vi "PPMS Interface.vi"() -> ()   [LabVIEW 2020]
uses:
  <vilib>/Analysis/1siggen.llb/Ramp Pattern by Samples.vi
  <vilib>/Utility/file.llb/Write Delimited Spreadsheet (string).vi
  <vilib>/Utility/file.llb/Write Delimited Spreadsheet (DBL).vi
  <vilib>/Analysis/NI_AALBase.lvlib
panel:
  out "IV Data":dbl[][](array[numeric])
  in  "scan_npts":i16
  out "scan_points":dbl[](array[numeric])
  out "scan_RATE":dbl=20.0
  out "scan_counter":i16=1000
  out "scan_head":i32=55
  out "scan_new":bool caption="Scan New"
  out "scan_env":string="MEASURE"
  out "Seq Line Now":i32=55
  out "AC Flag":bool caption="AC Current"
  in  "Filetype":u16(ring)=2 items=[".xlsx", ".txt", ".csv"]
  out "Wait Done":dbl=10.0
  in  "Measurement setup tabs":enum32{"DC Setup", "AC Setup", "I-V Setup"}(tab)=enum."AC Setup"
  in  "DC Pulse":bool=TRUE caption="Current Pulsing"
  in  "Channel 2":bool
  in  "Channel 1":bool=TRUE
  in  "Current Amplitude":string="1e-4"
  in  "Time Period (s)":string="3"
  in  "Tpad(ms)":i32=200
  in  "Voltmeter Range (V)":string="0.01"
  in  "NPLC":string="1"
  in  "Voltmeter Buffer Size":string="62"
  in  "Voltmeter 2 Address":string="8"
  in  "Voltmeter 1 Address":string="7"
  in  "6221 Address":string="12"
  in  "Configure DC System":bool
  in  "6221 Address 2":string="12" caption="6221 Address"
  in  "Current Amplitude 2":string="1e-4" caption="Current \nAmplitude"
  in  "Ch2 Enable":bool
  in  "Ch1 Enable":bool=TRUE
  in  "Buffer Data":enum16{"X", "XY", "RT", "XYRT"}(ring)=enum."RT"
  in  "Rate decimation":i32=2
  in  "SR860 Ch2 Address":string="5"
  in  "SR860 Ch1 Address":string="4"
  in  "Frequency":string="1711"
  in  "Filter BW":T1(ring)=enum."100ms"
  in  "Ch1 Harmonic":T2(ring)
  in  "Buffer Size (kB)":i32=2
  in  "Configure AC System":bool
  in  "Buffer Offset (kb)":string="0"
  in  "Ch2 Harmonic":T2(ring)
  in  "IV Datafile Root":path=path "C:/Users/QDUser/Desktop/LabVIEW Programs/PPMS Interface/testfiles/data/DC_IV_test"
  in  "SR860 Address - IV":string="4" caption="SR860 Address"
  in  "6221 Address - IV":string="12" caption="6221 Address"
  in  "IV Sampling":enum16{"Linear", "Logartihmic"}(ring)=enum."Logartihmic"
  in  "IV Type":T3(ring)
  in  "dI or Imin":dbl=1e-08
  in  "Imax":dbl=0.0001
  in  "Points":i16=17
  in  "2182A Address - IV":string="7" caption="2182A Address"
  in  "IV - DC/AC":bool=TRUE
  in  "DC Period (s)":string="0.5" caption="6221 Address"
  in  "2182A Buffer":string="11" caption="6221 Address"
  in  "Ch1 Harmonic - IV":T2(ring) caption="Harmonic"
  in  "Frequency - IV":string="1711" caption="Frequency"
  in  "Filter BW - IV":T4(ring)=enum."10 ms" caption="Filter BW"
  in  "Measurement \nSetup":u16(ring)=1 items=["DC Setup", "AC Setup", "I-V Setup"]
  in  "Measure Device":bool caption="Measure \nDevice"
  in  "Y-axis":u16(ring)=6 items=["Serial Number", "Time Elapsed (s)", "Temperature (K)", "Field (Oe)", "Theta (degree)", "Current excitation (A)", "Resistance 1 (ohm)", "STD 1 (ohm)", "Resistance 2 (ohm)", "STD 2 (ohm)", "Phase 1 (degrees)", "Phase 2 (degrees)"]
  in  "X-axis":u16(ring)=1 items=["Serial Number", "Time Elapsed (s)", "Temperature (K)", "Field (Oe)", "Theta (degree)", "Current excitation (A)", "Resistance 1 (ohm)", "STD 1 (ohm)", "Resistance 2 (ohm)", "STD 2 (ohm)", "Phase 1 (degrees)", "Phase 2 (degrees)"]
  out "XY Graph":cluster{"Data array":dbl[], "Data array":dbl[]}(graph)={"Data array"=[1000.1076049804688, 1000.095458984375, 1000.1318969726562, 999.822021484375, 916.6700439453125, 830.8634643554688, 742.8192749023438, 654.9420776367188, 567.0899047851562, 479.1545104980469, 392.864013671875, 304.93212890625, 216.95523071289062, 129.0848846435547, 41.132198333740234, -44.77364730834961, -132.77415466308594, -218.81509399414062, -306.63739013671875, -394.50677490234375, -482.4195251464844, -570.4457397460938, -658.3638305664062, -744.2162475585938, -832.0615234375, -920.28857421875, -999.9136352539062, -999.8893432617188, -999.877197265625, -966.5936279296875, -880.3653564453125, -790.4647827148438, -704.466064453125, -616.628173828125, -528.7174682617188, -442.6363525390625, -352.7901916503906, -266.7317810058594, -178.9671173095703, -91.0753402709961, -3.042452096939087, 84.87220001220703, 170.94114685058594, 258.7779235839844, 346.6785583496094, 434.949462890625, 520.9051513671875, 608.9139404296875, 696.776611328125, 782.679931640625, 870.5813598632812, 958.4483642578125, 1000.1197509765625, 1000.095458984375], "Data array"=[2.0974435134090905, 2.0958316086363635, 2.0992071125, 2.0990977595454545, 2.107740888863636, 2.1053484827272726, 2.1082263649999997, 2.1037182222727275, 2.083242016590909, 2.081601890227273, 2.0829138438636363, 2.0798880874999996, 2.0791002761363635, 2.0677500127272728, 1.8619974204545455, 1.1222847387045454, 0.8201078938409091, 0.7255154414090907, 0.6976336516363636, 0.7003691852045455, 0.6927557248181818, 0.7014058921818181, 0.6990065759090907, 0.7079667083181819, 0.7010926857727272, 0.6957325292954544, 0.6955325533636365, 0.697872530181818, 0.711508848840909, 0.7229268473181818, 0.7067185125454545, 0.6959014081136364, 0.6962725788181818, 0.7031570712499998, 0.6892584726363638, 0.6798120112272727, 0.6948854190227274, 0.70866324875, 0.7220332009318181, 0.7281562234318182, 1.006325211, 1.7135642684090908, 1.949954792045455, 2.0590681531818182, 2.084260665, 2.087814913863636, 2.0882882709090906, 2.090093333181818, 2.0964560554545457, 2.1017757368181815, 2.103902046363636, 2.0958079104545453, 2.1060686974999996, 2.0965902061363635]}
  out "WAIT delay(s)":u32=10
  out "Data array":dbl[][](array[numeric])
  out "Time Elasped":dbl format="%#_13g"
  out "Serial Number":i32=23
  out "Current StartTime":timestamp=timestamp(3802691718.054652 s since 1904-01-01)
  out "Current Filename":path=path "C:/Users/qmgmit/Desktop/Shivam/data/FGaT-WTe2/20230715_FGaT-WTe2_chip3_D1/test_sweep_0715_1929.csv"
  in  "Metadata":string="***** Metadata *****\nSample Description: Dummy\nCreator: Shivam\n"
  out "SET Rate":dbl=20.0
  out "SET Setpoint":dbl=1000.0
  out "Current Line Number":i32=10
  out "Parameters":dbl[][](array[numeric])
  out "ENV VAR":string="MEASURE"
  out "Current Line":string="STOP MEASURE "
  out "Command":string="STOP"
  in  "Datafile Path":path=path "C:/Users/QDUser/Desktop/LabVIEW Programs/PPMS External Control/testfiles/data/test_datafile_00_0602_1858.txt"
  out "Line Count":i32=10
  out "Array of commands":string[][](array[string])=[["## Field sweep to test device health"], ["NEWFILE test_sweep"], [""], ["START MEASURE"], ["WAIT MEASURE 10"], ["SET FIELD -1000 RATE 20"], ["WAIT FIELD 10"], ["SET FIELD 1000 RATE 20"], ["WAIT FIELD 10"], ["STOP MEASURE "]]
  out "Sequence File":string="## Field sweep to test device health\nNEWFILE test_sweep\n\nSTART MEASURE\nWAIT MEASURE 10\nSET FIELD -1000 RATE 20\nWAIT FIELD 10\nSET FIELD 1000 RATE 20\nWAIT FIELD 10\nSTOP MEASURE "
  in  "Sequence File":path=path "C:/Users/QDUser/Desktop/LabVIEW Programs/PPMS Interface/testfiles/seq/test_scan.lseq"
  out "STOP Flag":bool=TRUE
  out "Measure Blink":bool
  in  "Stop sequence":bool
  in  "Start Sequence":bool caption="Set Temperature"
  out "ExecSeq":bool caption="Executing Sequence"
  out "Measure Flag":bool caption="Measurement in progress"
  out "Field\nStatus":i32(ring)=4 items=["MagnetUnknown"=0, "StablePersistent"=1, "WarmingSwitch"=2, "CoolingSwitch"=3, "StableDriven"=4, "Iterating"=5, "Charging"=6, "Discharging"=7, "CurrentError"=8, "MagnetFailure"=15]
  out "Temperature\nStatus":i32(ring)=1 items=["TemperatureUnknown"=0, "Stable"=1, "Tracking"=2, "Near"=5, "Chasing"=6, "Filling"=7, "Standby"=10, "Disabled"=13, "ImpedanceNotFunction"=14, "TempFailure"=15]
  out "Chamber\nStatus":i32(ring)=1 items=["ChamberUnknown"=0, "PurgedAndSealed"=1, "VentedAndSealed"=2, "Sealed"=3, "Purging"=4, "Venting"=5, "PreHiVac"=6, "HighVac"=7, "PumpContinuous"=8, "VentContinuous"=9, "ChamberFailure"=15]
  out "Initialised":bool=TRUE
  in  "STOP Button":bool=TRUE
  in  "Set Chamber":bool caption="Set Temperature"
  in  "Set Position":bool caption="Set Temperature"
  in  "Set Field":bool caption="Set Temperature"
  in  "Set Temperature":bool
  in  "Chamber Setpoint":i32(ring)=5 caption="Chamber" items=["Seal", "PurgeAndSeal", "VentAndSeal", "PumpContinuous", "VentContinuous", "HighVacuum"]
  out "Theta":dbl=1.5735626220703125e-05 caption="Position"
  in  "Theta Setpoint":dbl caption="Theta (degrees)" min=-10.0 max=370.0
  out "Field":dbl=-0.10863074660301208
  out "Temperature":dbl=299.9990539550781
  in  "Field Setpoint":dbl=1000.0 caption="Field (Oe)" min=-90000.0 max=90000.0
  in  "Temperature setpoint":dbl=300.0 caption="Temperature (K)" min=1.8 max=400.0
  in  "InstrumentType":i32(ring)=2 items=["PPMS", "VersaLab", "DynaCool", "SVSM", "OptiCool"]
  in  "Remote \nMode":bool
  in  "IP Address":string="10.29.168.8"
  # "AC IV"
  # "DC IV"
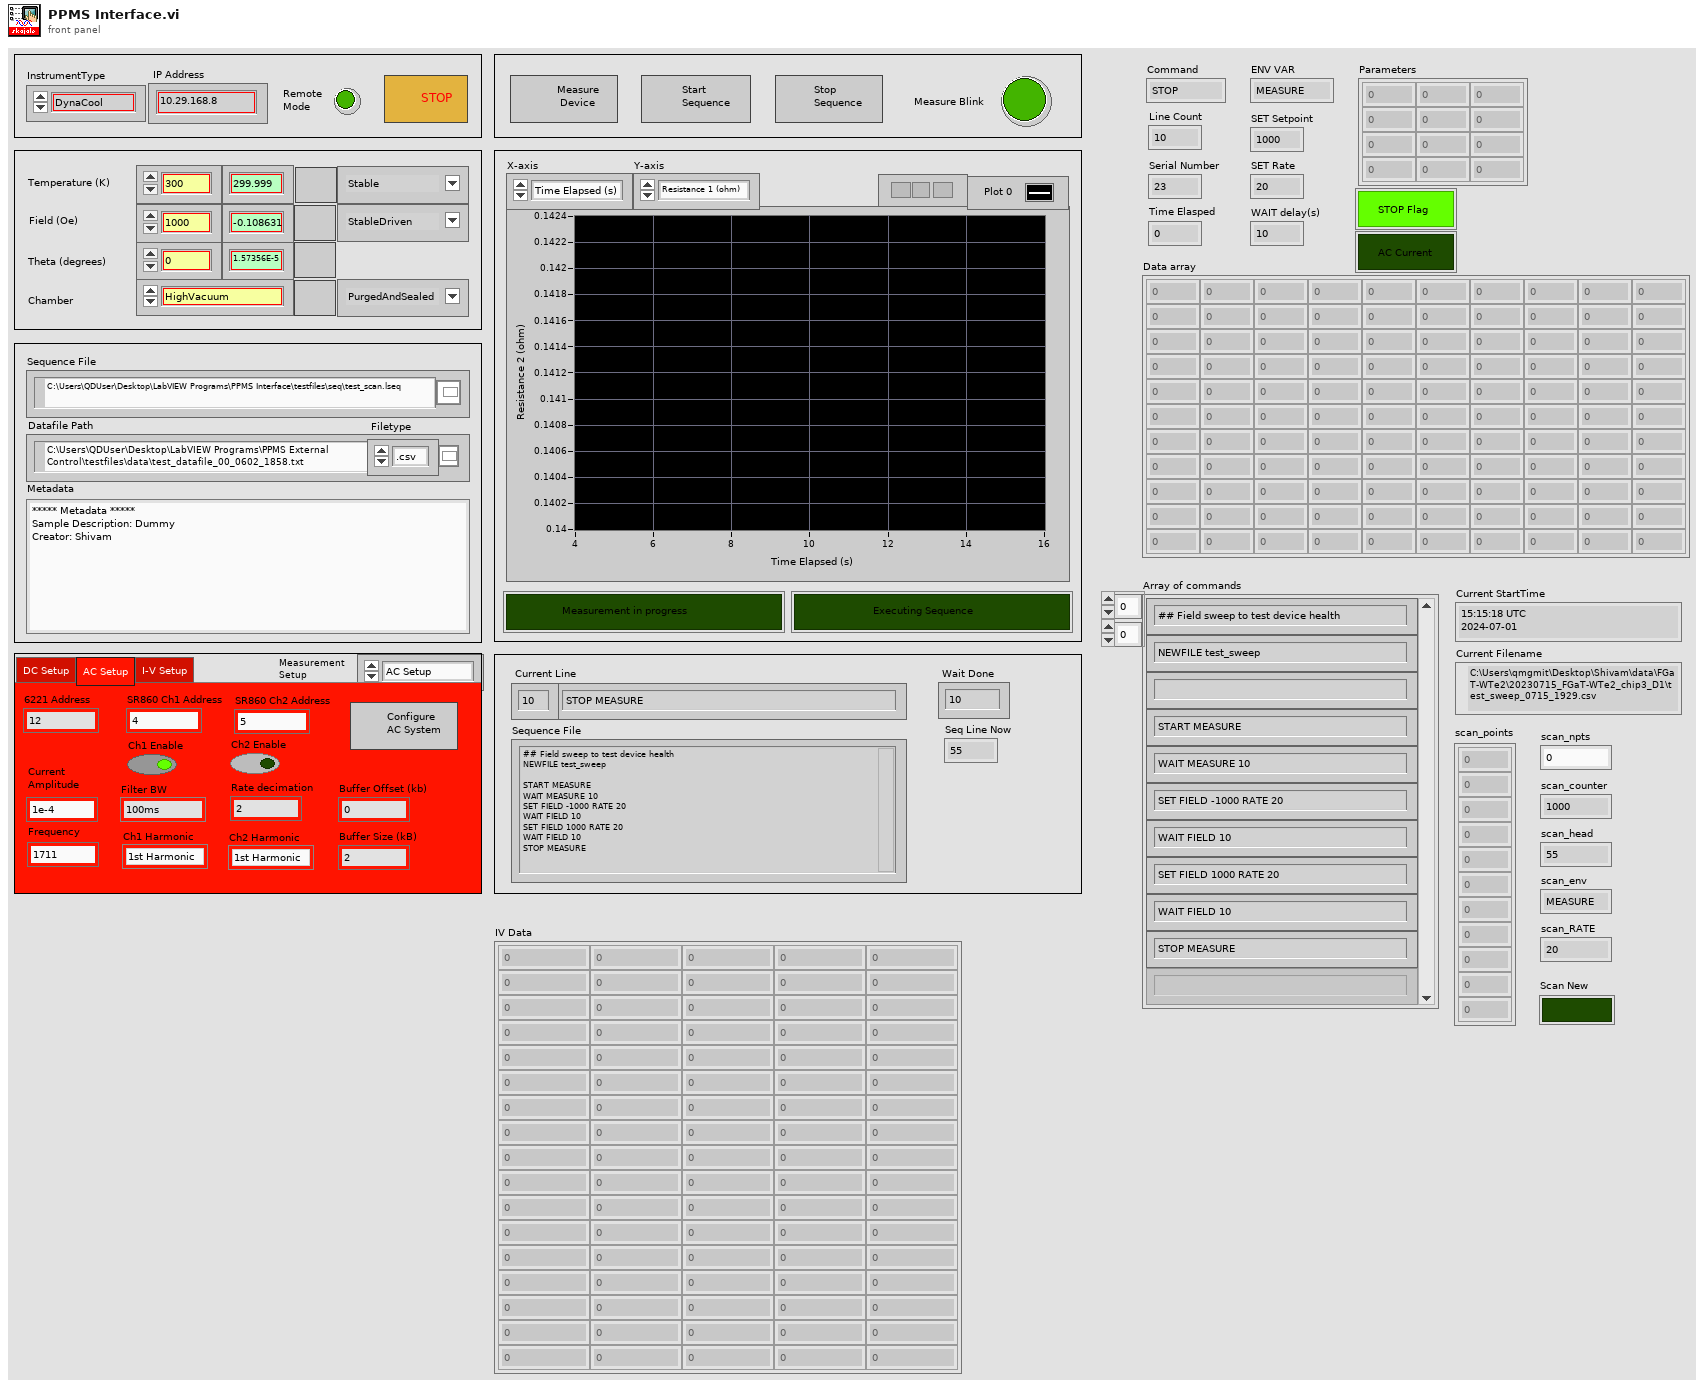
[diagram p1: front panel]
types:
  T1 = enum16{"1us", "3us", "10us", "30us", "100us", "300us", "1ms", "3ms", "10ms", "30ms", "100ms", "300ms", "1s"}
  T2 = enum16{"1st Harmonic", "2nd Harmonic", "3rd Harmonic"}
  T3 = enum16{"0 : Imax", "0 : Imax : 0", "0 : Imax : -Imax : 0", "-Imax : 0 : Imax"}
  T4 = enum16{"1 us", "3 us", "10 us", "30 us", "100 us", "300 us", "1 ms", "3 ms", "10 ms", "30 ms", "100 ms", "300 ms", "1 s", "3 s", "10 s", "30 s", "100 s", "300 s"}
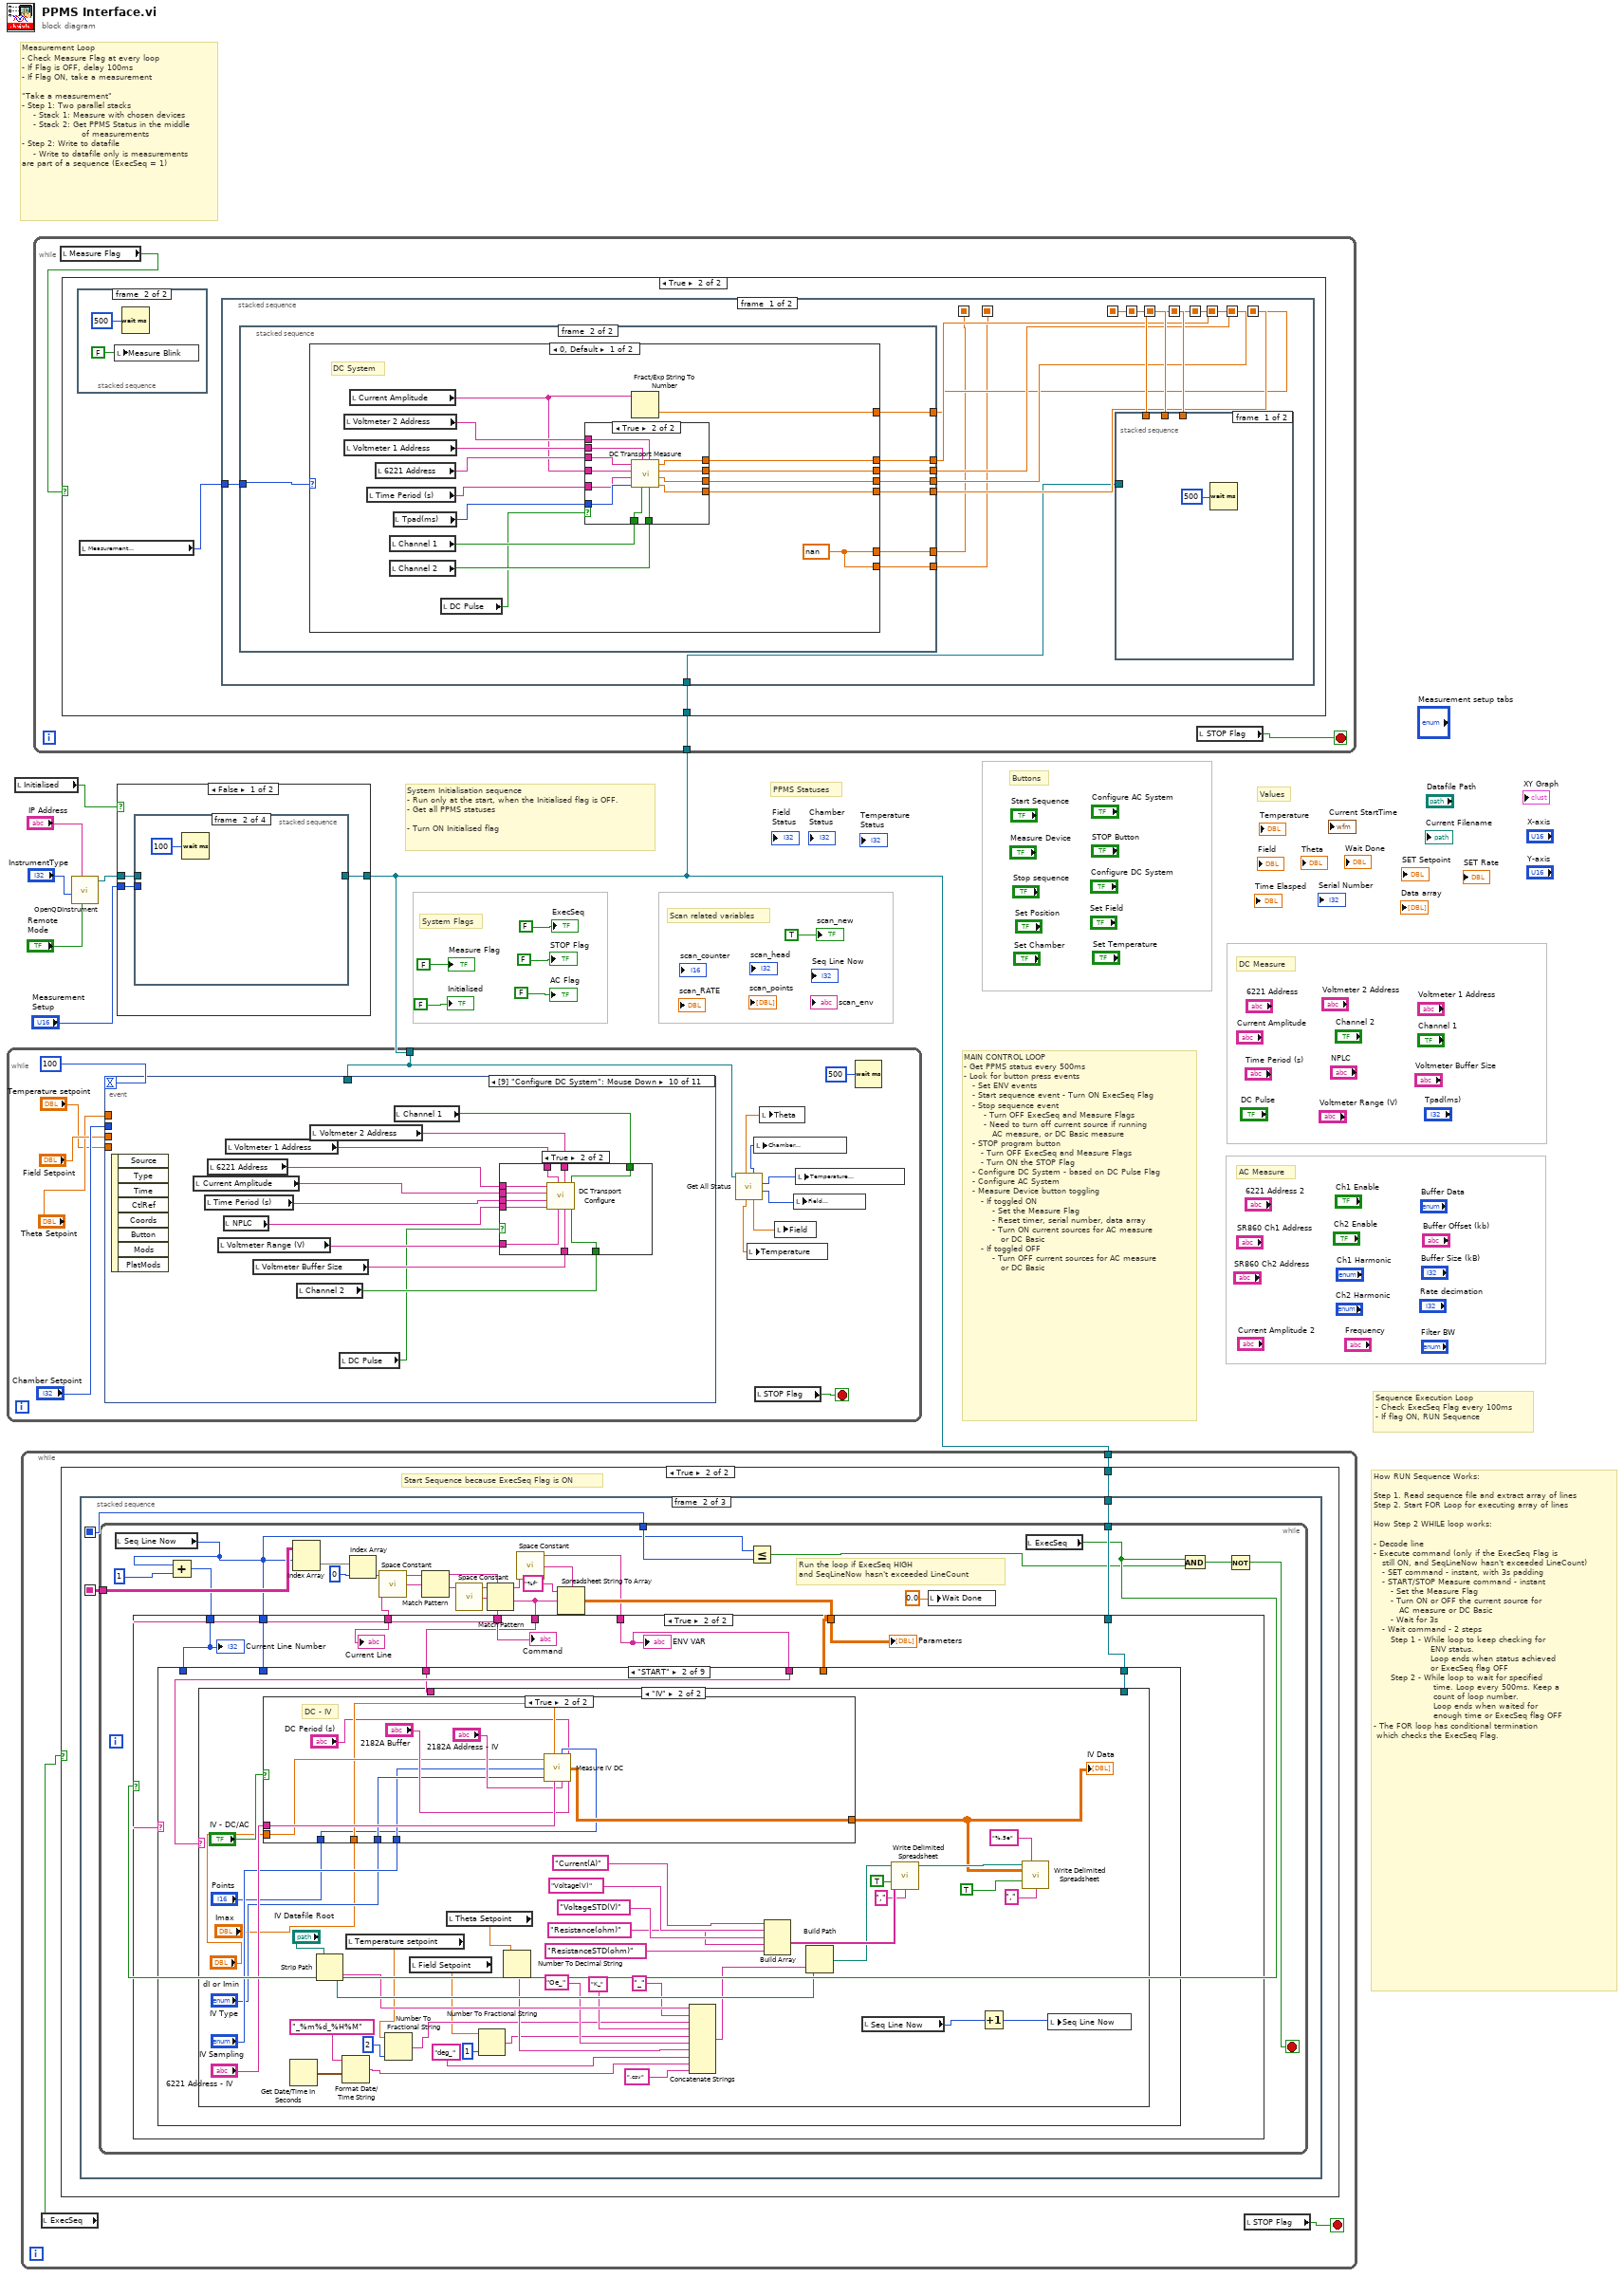
[diagram p0: block diagram]
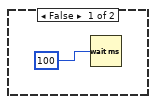
[diagram p2: hidden frame]
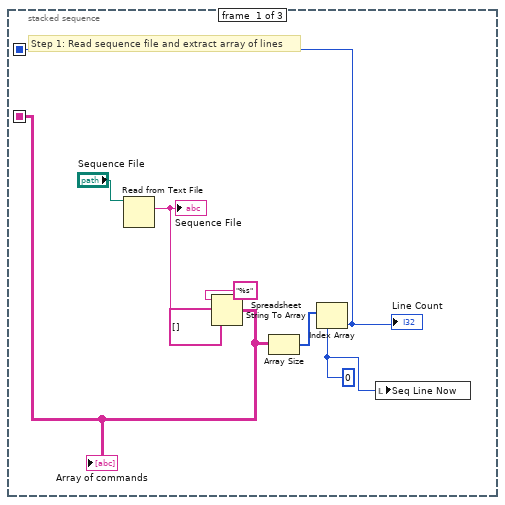
[diagram p3: hidden frame]
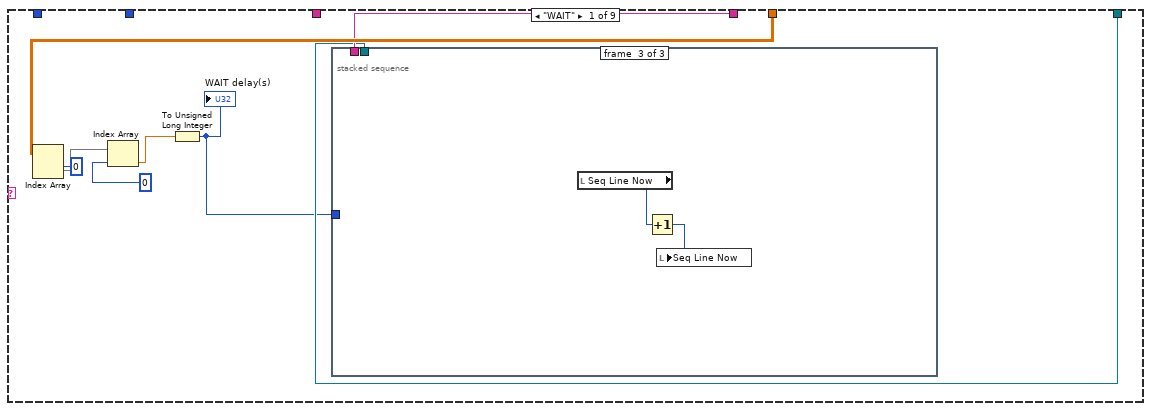
[diagram p5: hidden frame]
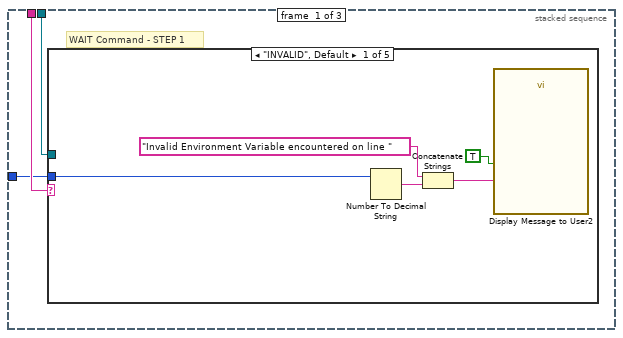
[diagram p6: hidden frame]
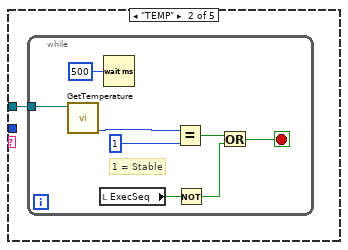
[diagram p7: hidden frame]
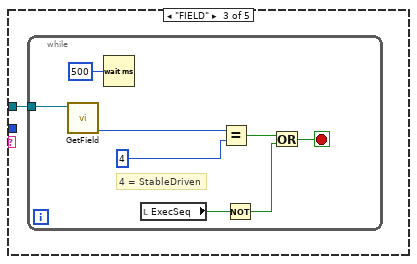
[diagram p8: hidden frame]
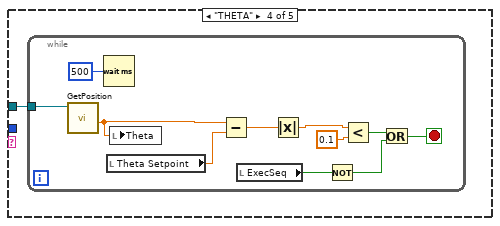
[diagram p9: hidden frame]
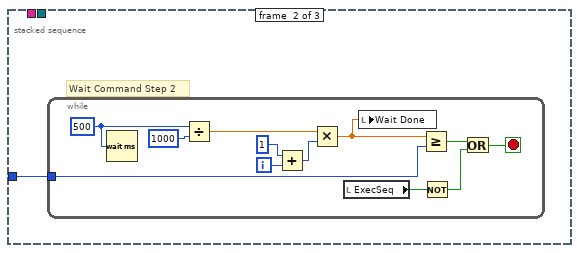
[diagram p11: hidden frame]
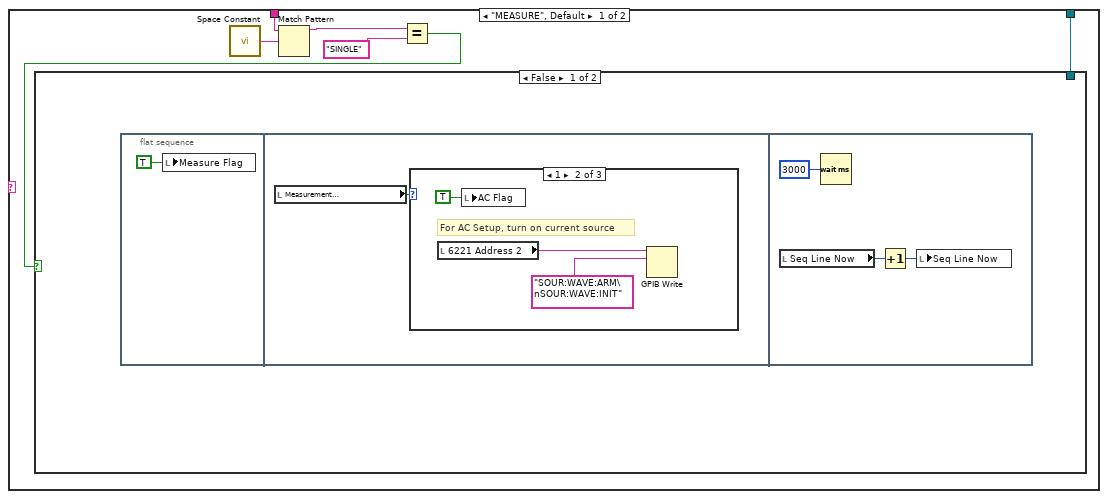
[diagram p12: hidden frame]
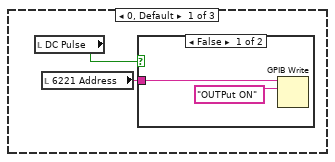
[diagram p13: hidden frame]
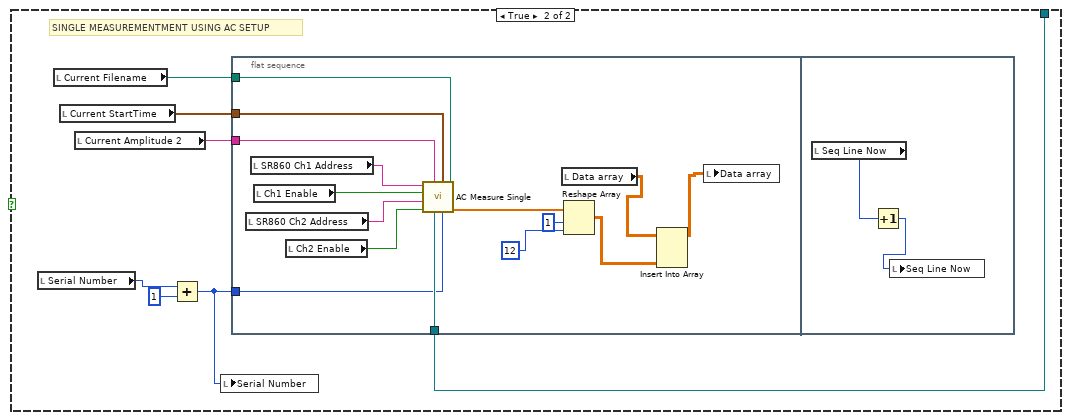
[diagram p16: hidden frame]
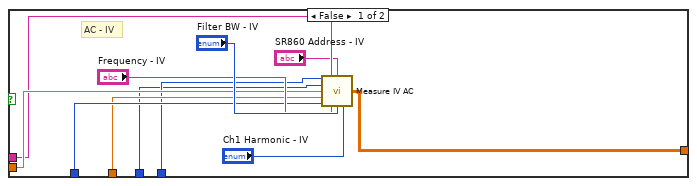
[diagram p17: hidden frame]
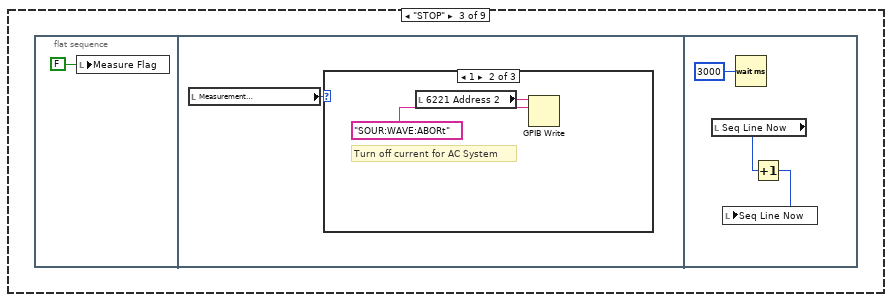
[diagram p18: hidden frame]
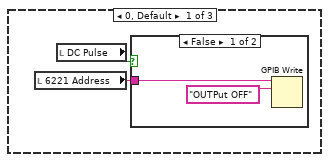
[diagram p19: hidden frame]
diagram:
  # "Scan related variables"
  # "AC Measure"
  # "DC Measure"
  # "How RUN Sequence Works:\n\nStep 1. Read sequence file and extract array of lines \nStep 2. Start FOR Loop for executing array of lines\n\nHow Step 2 WHILE loop works:\n\n- Decode line\n- Execute command (only if the ExecSeq Flag is \n   still ON, and SeqLineNow hasn't exceeded LineCount)\n   - SET command - instant, with 3s padding\n   - START/STOP Measure command - instant\n      - Set the Measure Flag\n      - Turn ON or OFF the current source for \n         AC measure or DC Basic\n      - Wait for 3s\n   - Wait command - 2 steps\n      Step 1 - While loop to keep checking for\n                    ENV status.\n                    Loop ends when status achieved \n                    or ExecSeq flag OFF\n      Step 2 - While loop to wait for specified \n                     time. Loop every 500ms. Keep a \n                     count of loop number.\n                     Loop ends when waited for \n                     enough time or ExecSeq flag OFF\n- The FOR loop has conditional termination\n which checks the ExecSeq Flag."
  # "Sequence Execution Loop\n- Check ExecSeq Flag every 100ms\n- If flag ON, RUN Sequence"
  # "MAIN CONTROL LOOP\n- Get PPMS status every 500ms\n- Look for button press events\n   - Set ENV events\n   - Start sequence event - Turn ON ExecSeq Flag\n   - Stop sequence event \n       - Turn OFF ExecSeq and Measure Flags\n       - Need to turn off current source if running\n          AC measure, or DC Basic measure\n   - STOP program button \n      - Turn OFF ExecSeq and Measure Flags\n      - Turn ON the STOP Flag\n   - Configure DC System - based on DC Pulse Flag\n   - Configure AC System\n   - Measure Device button toggling\n      - If toggled ON \n          - Set the Measure Flag\n          - Reset timer, serial number, data array\n          - Turn ON current sources for AC measure \n             or DC Basic\n      - If toggled OFF\n          - Turn OFF current sources for AC measure \n             or DC Basic"
  # "System Flags"
  # "PPMS Statuses"
  # "Values"
  # "Buttons"
  # "System Initialisation sequence\n- Run only at the start, when the Initialised flag is OFF.\n- Get all PPMS statuses\n\n- Turn ON Initialised flag"
  # "Measurement Loop\n- Check Measure Flag at every loop\n- If Flag is OFF, delay 100ms\n- If Flag ON, take a measurement\n\n\"Take a measurement\"\n- Step 1: Two parallel stacks\n    - Stack 1: Measure with chosen devices\n    - Stack 2: Get PPMS Status in the middle\n                     of measurements\n- Step 2: Write to datafile\n    - Write to datafile only is measurements    are part of a sequence (ExecSeq = 1)"
  n1 = local read "Initialised"() -> (w9:bool)
  n2 = call "OpenQDInstrument.vi"("Remote"="Remote \nMode", "IP Address"="IP Address", "InstrumentType"="InstrumentType") -> ("Instrument Ref"=w8:refnum<k24>)  [unwired: 5 in, 1 out]
  n3 = case shown="False" w9 {
    tunnel: w8 -> [w16 w27]
    tunnel: [w15 w27] -> w4
    tunnel: "Measurement \nSetup" -> [w14 _]
    frame False {
      n4 = stacked-sequence {
        tunnel: w16 -> [w24 _ _ _]
        tunnel: [w18 _ _ _] -> w15
        tunnel: w14 -> [_ _ _ _]
        frame #0 {
          n5 = call "Get All Status.vi"("Instrument Ref In"=w24) -> ("Field\nStatus"=w21:i32, "Temperature\nStatus"=w22:i32, "Instrument Ref Out"=w18:refnum<k24>, "Field"=w19:dbl, "Chamber\nStatus"=w23:i32, "Temperature"=w20:dbl, "Position"=w17:dbl)  [unwired: 3 in, 1 out]
          n6 = local write "Theta"(w17) -> ()
          n7 = local write "Chamber\nStatus"(w23) -> ()
          n8 = local write "Temperature\nStatus"(w22) -> ()
          n9 = local write "Field\nStatus"(w21) -> ()
          n10 = local write "Field"(w19) -> ()
          n11 = local write "Temperature"(w20) -> ()
        }
        frame #1 {
          n12 = Wait (ms)(milliseconds to wait=u32 100) -> ()  [unwired: 1 out]
        }
        frame #2 {
        }
        frame #3 {
          n13 = local write "Initialised"(TRUE ("Initialised")) -> ()
        }
      }
    }
    frame True {
    }
  }
  n14 = while {
    tunnel: w4 -> [w32]
    stop <- w29 stop-if-true
    n15 = event shown="[9] \"Configure DC System\": Mouse Down" {
      selector: _ -> [_ _ _ _ _ _ _ _ _ _ _]
      dyn-events: _ -> [_ _ _ _ _ _ _ _ _ _ _]
      timeout: 100 -> [_ _ _ _ _ _ _ _ _ _ _]
      tunnel: "Chamber Setpoint" -> [_ _ w73 _ _ _ _ _ _ _ _]
      tunnel: w32 -> [_ _ w72 w77 w79 w83 _ _ _ _ _]
      tunnel: "Temperature setpoint" -> [_ _ _ w74 _ _ _ _ _ _ _]
      tunnel: "Field Setpoint" -> [_ _ _ _ w78 _ _ _ _ _ _]
      tunnel: "Theta Setpoint" -> [_ _ _ _ _ w82 _ _ _ _ _]
      event Timeout {
        # "Use timeout to update graph"
        n16 = event-data() -> ()  [unwired: 1 in, 3 out]
        n17 = local read "Data array"() -> (w49:dbl[][])
        n18 = property on="Y-axis" class="Ring (strict)"() -> ("RingText.Text"=w42:string)  [unwired: 2 in, 2 out]
        n19 = property on="X-axis" class="Ring (strict)"() -> ("RingText.Text"=w43:string)  [unwired: 2 in, 2 out]
        n20 = local read "Y-axis"() -> (w45:u16)
        n21 = local read "X-axis"() -> (w46:u16)
        n22 = Index Array(array=w49, index (col) #1=w46, index (col) #2=w45) -> (element #1=w48:dbl[], element #2=w47:dbl[])  [unwired: 2 in]
        n23 = Bundle("Data array"=w48, "Data array"=w47) -> (w44:cluster{"Data array":dbl[], "Data array":dbl[]})  [unwired: 1 in]
        n24 = property on="XY Graph" class="XYGraph (strict)"("XScale.NameLbl.Text"=w43, "YScale.NameLbl.Text"=w42) -> ()  [unwired: 2 in, 2 out]
        n25 = local write "XY Graph"(w44) -> ()
      }
      event "Measure Device": Value Change {
        n26 = event-data() -> ()  [unwired: 1 in, 6 out]
        n27 = local read "Measure Device"() -> (w50:bool)
        n28 = case shown="True" w50 {
          frame False {
            n29 = local read "Measurement \nSetup"() -> (w51:u16)
            n30 = case shown="0, Default" w51 {
              frame 0, Default {
                # "Turn off 6221 if DC Basic"
                n31 = local read "6221 Address"() -> (w52:string)
                n32 = local read "DC Pulse"() -> (w53:bool)
                n33 = case shown="False" w53 {
                  tunnel: w52 -> [w54 _]
                  frame False {
                    n34 = GPIB Write(0:w54, 1:"OUTPut OFF" ("data")) -> ()  [unwired: 3 in, 2 out]
                  }
                  frame True {
                  }
                }
              }
              frame 1 {
                # "Turn off 6221 for AC System"
                n35 = local read "6221 Address 2"() -> (w56:string)
                n36 = GPIB Write(0:w56, 1:"SOUR:WAVE:ABORt" ("data")) -> ()  [unwired: 3 in, 2 out]
              }
              frame 2 {
              }
            }
          }
          frame True {
            n37 = Get Date/Time In Seconds() -> (seconds since 1Jan1904=w59:timestamp)
            n38 = local write "Time Elasped"(0.0 ("Time Elasped")) -> ()
            n39 = local write "Serial Number"(0 ("Serial Number")) -> ()
            n40 = local read "Measurement \nSetup"() -> (w58:u16)
            n41 = local write "Current StartTime"(w59) -> ()
            n42 = local write "Data array"(dbl[][] [] ("Data array")) -> ()
            n43 = case shown="0, Default" w58 {
              frame 0, Default {
                n44 = local read "6221 Address"() -> (w63:string)
                n45 = local read "DC Pulse"() -> (w64:bool)
                n46 = case shown="False" w64 {
                  tunnel: w63 -> [w66 _]
                  frame False {
                    n47 = Wait (ms)(milliseconds to wait=u32 1000) -> ()  [unwired: 1 out]
                    n48 = GPIB Write(0:w66, 1:"OUTPut ON" ("data")) -> ()  [unwired: 3 in, 2 out]
                  }
                  frame True {
                  }
                }
              }
              frame 1 {
                n49 = local read "6221 Address 2"() -> (w70:string)
                n50 = local write "AC Flag"(TRUE ("AC Flag")) -> ()
                n51 = Wait (ms)(milliseconds to wait=u32 1000) -> ()  [unwired: 1 out]
                n52 = GPIB Write(0:w70, 1:"SOUR:WAVE:ARM\nSOUR:WAVE:INIT" ("data")) -> ()  [unwired: 3 in, 2 out]
              }
              frame 2 {
              }
            }
          }
        }
        n53 = local write "Measure Flag"(w50) -> ()
      }
      event "Set Chamber": Mouse Down {
        n54 = event-data() -> ()  [unwired: 1 in, 8 out]
        n55 = call "SetChamber.vi"("Code"=w73, "Instrument Ref In"=w72) -> ()  [unwired: 1 in, 3 out]
      }
      event "Set Temperature": Mouse Down {
        w75 = 0 items=["FastSettle", "NoOvershoot"] ("Approach")
        n56 = event-data() -> ()  [unwired: 1 in, 8 out]
        n57 = call "SetTemperature.vi"("Approach"=w75, "Rate"=10.0, "Temperature"=w74, "Instrument Ref In"=w77) -> ()  [unwired: 3 in, 3 out]
      }
      event "Set Field": Mouse Down {
        n58 = event-data() -> ()  [unwired: 1 in, 8 out]
        n59 = call "SetField.vi"("Rate"=200.0, "Field"=w78, "Instrument Ref In"=w79) -> ()  [unwired: 4 in, 3 out]
      }
      event "Set Position": Mouse Down {
        n60 = event-data() -> ()  [unwired: 1 in, 8 out]
        n61 = call "SetPosition.vi"("Speed"=2.0, "Position"=w82, "Instrument Ref In"=w83) -> ()  [unwired: 4 in, 3 out]
      }
      event "Start Sequence": Mouse Down {
        n62 = event-data() -> ()  [unwired: 1 in, 8 out]
        n63 = local write "ExecSeq"(TRUE ("ExecSeq")) -> ()
      }
      event "Stop sequence": Mouse Down {
        w86 = FALSE ("ExecSeq")
        n64 = event-data() -> ()  [unwired: 1 in, 8 out]
        n65 = local read "Measurement \nSetup"() -> (w85:u16)
        n66 = local write "Measure Flag"(w86) -> ()
        n67 = local write "ExecSeq"(w86) -> ()
        n68 = case shown="1" w85 {
          frame 0, Default {
            n69 = local read "6221 Address"() -> (w87:string)
            n70 = local read "DC Pulse"() -> (w88:bool)
            n71 = case shown="False" w88 {
              tunnel: w87 -> [w89 _]
              frame False {
                n72 = GPIB Write(0:w89, 1:"CURR OFF" ("data")) -> ()  [unwired: 3 in, 2 out]
              }
              frame True {
              }
            }
          }
          frame 1 {
            n73 = local read "6221 Address 2"() -> (w92:string)
            n74 = GPIB Write(0:w92, 1:"SOUR:WAVE:ABORt" ("data")) -> ()  [unwired: 3 in, 2 out]
          }
          frame 2 {
          }
        }
      }
      event "STOP Button": Mouse Down {
        n75 = event-data() -> ()  [unwired: 1 in, 8 out]
        n76 = stacked-sequence {
          frame #0 {
            w93 = FALSE ("Measure Flag")
            n77 = local write "ExecSeq"(w93) -> ()
            n78 = local write "Measure Flag"(w93) -> ()
          }
          frame #1 {
            n79 = Wait (ms)(milliseconds to wait=u32 1000) -> ()  [unwired: 1 out]
          }
          frame #2 {
            n80 = local write "STOP Flag"(TRUE ("STOP Flag")) -> ()
          }
        }
      }
      event "Configure DC System": Mouse Down {
        n81 = event-data() -> ()  [unwired: 1 in, 8 out]
        n82 = local read "Current Amplitude"() -> (w97:string)
        n83 = local read "Time Period (s)"() -> (w98:string)
        n84 = local read "6221 Address"() -> (w103:string)
        n85 = local read "Voltmeter Range (V)"() -> (w100:string)
        n86 = local read "NPLC"() -> (w99:string)
        n87 = local read "Voltmeter 1 Address"() -> (w104:string)
        n88 = local read "Voltmeter Buffer Size"() -> (w101:string)
        n89 = local read "Channel 2"() -> (w102:bool)
        n90 = local read "Voltmeter 2 Address"() -> (w105:string)
        n91 = local read "DC Pulse"() -> (w96:bool)
        n92 = local read "Channel 1"() -> (w106:bool)
        n93 = case shown="True" w96 {
          tunnel: w106 -> [w115 w125]
          tunnel: w105 -> [w114 w124]
          tunnel: w104 -> [w113 w123]
          tunnel: w103 -> [w112 w122]
          tunnel: w102 -> [w108 w121]
          tunnel: w101 -> [w107 w120]
          tunnel: w100 -> [w109 w119]
          tunnel: w99 -> [w110 w118]
          tunnel: w98 -> [_ w117]
          tunnel: w97 -> [w111 w116]
          frame False {
            n94 = call "DC Basic Configure.vi"("Channel 2"=w108, "Channel 1"=w115, "Voltmeter Buffer Size"=w107, "Voltmeter 2 Address"=w114, "Voltmeter Range (V)"=w109, "Voltmeter 1 Address"=w113, "NPLC"=w110, "Current Amplitude"=w111, "6221 Address"=w112) -> ()  [unwired: 3 in]
          }
          frame True {
            n95 = call "DC Transport Configure.vi"("Channel 2"=w121, "Channel 1"=w125, "Voltmeter Buffer Size"=w120, "Voltmeter 2 Address"=w124, "Voltmeter Range (V)"=w119, "Voltmeter 1 Address"=w123, "NPLC"=w118, "Time Period (s)"=w117, "Current Amplitude"=w116, "6221 Address"=w122) -> ()  [unwired: 2 in]
          }
        }
      }
      event "Configure AC System": Mouse Down {
        n96 = event-data() -> ()  [unwired: 1 in, 8 out]
        n97 = local read "SR860 Ch1 Address"() -> (w132:string)
        n98 = local read "Current Amplitude 2"() -> (w134:string)
        n99 = local read "Buffer Size (kB)"() -> (w128:i32)
        n100 = local read "Ch1 Harmonic"() -> (w127:T2)
        n101 = local read "Frequency"() -> (w135:string)
        n102 = local read "Filter BW"() -> (w136:T1)
        n103 = local read "6221 Address 2"() -> (w133:string)
        n104 = local read "Ch2 Harmonic"() -> (w126:T2)
        n105 = local read "Ch1 Enable"() -> (w131:bool)
        n106 = local read "SR860 Ch2 Address"() -> (w130:string)
        n107 = local read "Rate decimation"() -> (w137:i32)
        n108 = local read "Ch2 Enable"() -> (w129:bool)
        n109 = call "AC Transport Configure.vi"("6221 Address"=w133, "SR860 Ch1 Address"=w132, "Ch1 Enable"=w131, "SR860 Ch2 Address"=w130, "Ch2 Enable"=w129, "Current Amplitude"=w134, "Frequency"=w135, "Filter BW"=w136, "Buffer Size (kB)"=w128, "Ch1 Harmonic"=w127, "Ch2 Harmonic"=w126, "Rate decimation"=w137) -> ()  [unwired: 1 in, 3 out]
      }
    }
    n110 = call "Get All Status.vi"("Instrument Ref In"=w32) -> ("Field\nStatus"=w36:i32, "Temperature\nStatus"=w35:i32, "Field"=w38:dbl, "Chamber\nStatus"=w34:i32, "Temperature"=w37:dbl, "Position"=w31:dbl)  [unwired: 3 in, 2 out]
    n111 = local write "Temperature"(w37) -> ()
    n112 = local write "Chamber\nStatus"(w34) -> ()
    n113 = local read "STOP Flag"() -> (w29:bool)
    n114 = local write "Theta"(w31) -> ()
    n115 = local write "Field"(w38) -> ()
    n116 = local write "Field\nStatus"(w36) -> ()
    n117 = local write "Temperature\nStatus"(w35) -> ()
    n118 = Wait (ms)(milliseconds to wait=u32 500) -> ()  [unwired: 1 out]
  }
  n119 = while {
    tunnel: w4 -> [w138]
    stop <- w140 stop-if-true
    n120 = local read "ExecSeq"() -> (w139:bool)
    n121 = case shown="True" w139 {
      tunnel: w138 -> [_ w142]
      frame False {
        n122 = Wait (ms)(milliseconds to wait=u32 100) -> ()  [unwired: 1 out]
      }
      frame True {
        # "Start Sequence because ExecSeq Flag is ON"
        n123 = stacked-sequence {
          seq-local: [w145 _ _] -> [_ w151 _]
          seq-local: [w144 _ _] -> [_ w153 _]
          tunnel: w142 -> [_ w152 _]
          frame #0 {
            w143 = 0 ("index")
            # "Step 1: Read sequence file and extract array of lines"
            n124 = Read from Text File(file (use dialog)="Sequence File") -> (text=w149:string)  [unwired: 3 in, 3 out]
            "Sequence File" <- w149
            n125 = Spreadsheet String To Array(format string="%s", spreadsheet string=w149, array type (2D Dbl)=string[][] []) -> (array=w144:string[][])  [unwired: 1 in]
            "Array of commands" <- w144
            n126 = Array Size(array=w144) -> (size(s)=w150:i32[])
            n127 = Index Array(array=w150, index=w143) -> (element=w145:i32)
            "Line Count" <- w145
            n128 = local write "Seq Line Now"(w143) -> ()
          }
          frame #1 {
            n129 = while {
              tunnel: w153 -> [w169]
              tunnel: w152 -> [w163]
              tunnel: w151 -> [w159]
              stop <- w162 stop-if-true
              # "Run the loop if ExecSeq HIGH\nand SeqLineNow hasn't exceeded LineCount"
              n130 = local read "Seq Line Now"() -> (w155:i32)
              n131 = Add(x=w155, y=1) -> (x+y=w161:i32)
              n132 = Index Array(array=w169, index (row)=w155) -> (element=w168:string[])  [unwired: 1 in]
              n133 = Index Array(array=w168, index=0) -> (element=w167:string)
              n134 = call <vilib>:"Space Constant.vi"() -> ("String"=w176:string)
              n135 = Match Pattern(string=w167, regular expression=w176) -> (before substring=w166:string, after substring=w174:string)  [unwired: 1 in, 2 out]
              n136 = call <vilib>:"Space Constant.vi"() -> ("String"=w173:string)
              n137 = Match Pattern(string=w174, regular expression=w173) -> (before substring=w164:string, after substring=w154:string)  [unwired: 1 in, 2 out]
              n138 = call <vilib>:"Space Constant.vi"() -> ("String"=w171:string)
              n139 = Spreadsheet String To Array(delimiter (Tab)=w171, format string="%f", spreadsheet string=w154) -> (array=w165:dbl[][])  [unwired: 1 in]
              n140 = Less Or Equal?(x=w155, y=w159) -> (x <= y?=w156:bool)
              n141 = local write "Wait Done"(0.0 ("Wait Done")) -> ()
              n142 = local read "ExecSeq"() -> (w157:bool)
              n143 = case shown="True" w157 {
                tunnel: w167 -> [_ w184]
                tunnel: w166 -> [_ w183]
                tunnel: w165 -> [_ w182]
                tunnel: w164 -> [_ w181]
                tunnel: w163 -> [_ w180]
                tunnel: w161 -> [_ w179]
                tunnel: w155 -> [_ w178]
                tunnel: w154 -> [_ w177]
                frame False {
                }
                frame True {
                  n144 = case shown="\"START\"" w183 {
                    tunnel: w182 -> [w188 _ _ w369 w448 _ _ _ w483]
                    tunnel: w181 -> [w187 w248 _ w368 _ w468 _ _ w480]
                    tunnel: w179 -> [_ _ _ w366 _ _ _ _ w479]
                    tunnel: w180 -> [w186 w246 _ w367 _ _ _ _ w478]
                    tunnel: w178 -> [_ _ _ w370 _ _ _ _ _]
                    tunnel: w177 -> [_ w247 _ _ _ _ _ _ _]
                    frame "WAIT" {
                      n145 = Index Array(array=w188, index (row)=0) -> (element=w189:dbl[])  [unwired: 1 in]
                      n146 = Index Array(array=w189, index=0) -> (element=w190:dbl)
                      n147 = To Unsigned Long Integer(number=w190) -> (unsigned 32bit integer=w185:u32)
                      "WAIT delay(s)" <- w185
                      n148 = stacked-sequence {
                        tunnel: w187 -> [w195 _ _]
                        tunnel: w185 -> [w194 w231 _]
                        tunnel: w186 -> [w193 _ _]
                        frame #0 {
                          # "WAIT Command - STEP 1"
                          n149 = case shown="\"INVALID\", Default" w195 {
                            tunnel: w194 -> [w197 _ _ _ _]
                            tunnel: w193 -> [_ w201 w210 w219 _]
                            frame "INVALID", Default {
                              n150 = Number To Decimal String(number=w197) -> (decimal integer string=w198:string)  [unwired: 1 in]
                              n151 = Concatenate Strings("Invalid Environment Variable encountered on line " ("string"), w198) -> (w196:string)
                              n152 = call "Display Message to User2"("Enable"=TRUE, "Message"=w196) -> ()  [unwired: 8 in, 2 out]
                            }
                            frame "TEMP" {
                              n153 = while {
                                tunnel: w201 -> [w202]
                                stop <- w203 stop-if-true
                                # "1 = Stable"
                                n154 = call "GetTemperature.vi"("Instrument Ref In"=w202) -> ("Temperature\nStatus"=w207:i32)  [unwired: 4 in, 4 out]
                                n155 = local read "ExecSeq"() -> (w206:bool)
                                n156 = Wait (ms)(milliseconds to wait=u32 500) -> ()  [unwired: 1 out]
                                n157 = Equal?(x=w207, y=1) -> (x = y?=w205:bool)
                                n158 = Not(x=w206) -> (.not. x?=w204:bool)
                                n159 = Or(x=w205, y=w204) -> (x .or. y?=w203:bool)
                              }
                            }
                            frame "FIELD" {
                              n160 = while {
                                tunnel: w210 -> [w212]
                                stop <- w213 stop-if-true
                                # "4 = StableDriven"
                                n161 = call "GetField.vi"("Instrument Ref In"=w212) -> ("Field\nStatus"=w216:i32)  [unwired: 4 in, 4 out]
                                n162 = Wait (ms)(milliseconds to wait=u32 500) -> ()  [unwired: 1 out]
                                n163 = local read "ExecSeq"() -> (w215:bool)
                                n164 = Equal?(x=w216, y=4) -> (x = y?=w214:bool)
                                n165 = Not(x=w215) -> (.not. x?=w211:bool)
                                n166 = Or(x=w214, y=w211) -> (x .or. y?=w213:bool)
                              }
                            }
                            frame "THETA" {
                              n167 = while {
                                tunnel: w219 -> [w225]
                                stop <- w220 stop-if-true
                                n168 = call "GetPosition.vi"("Instrument Ref In"=w225) -> ("Position"=w229:dbl)  [unwired: 3 in, 3 out]
                                n169 = Wait (ms)(milliseconds to wait=u32 500) -> ()  [unwired: 1 out]
                                n170 = local read "Theta Setpoint"() -> (w224:dbl)
                                n171 = local write "Theta"(w229) -> ()
                                n172 = Subtract(x=w229, y=w224) -> (x-y=w228:dbl)
                                n173 = local read "ExecSeq"() -> (w223:bool)
                                n174 = Absolute Value(x=w228) -> (abs(x)=w227:dbl)
                                n175 = Not(x=w223) -> (.not. x?=w222:bool)
                                n176 = Less?(x=w227, y=0.1) -> (x < y?=w221:bool)
                                n177 = Or(x=w221, y=w222) -> (x .or. y?=w220:bool)
                              }
                            }
                            frame "MEASURE" {
                            }
                          }
                        }
                        frame #1 {
                          # "Wait Command Step 2"
                          n178 = while {
                            tunnel: w231 -> [w233]
                            i -> [w242]
                            stop <- w237 stop-if-true
                            w241 = u32 500 ("milliseconds to wait")
                            n179 = Wait (ms)(milliseconds to wait=w241) -> ()  [unwired: 1 out]
                            n180 = Divide(x=w241, y=u32 1000) -> (x/y=w239:dbl)
                            n181 = Add(x=1, y=w242) -> (x+y=w235:i32)
                            n182 = Multiply(x=w239, y=w235) -> (x*y=w232:dbl)
                            n183 = local read "ExecSeq"() -> (w243:bool)
                            n184 = local write "Wait Done"(w232) -> ()
                            n185 = Greater Or Equal?(x=w232, y=w233) -> (x >= y?=w238:bool)
                            n186 = Not(x=w243) -> (.not. x?=w236:bool)
                            n187 = Or(x=w238, y=w236) -> (x .or. y?=w237:bool)
                          }
                        }
                        frame #2 {
                          n188 = local read "Seq Line Now"() -> (w244:i32)
                          n189 = Increment(x=w244) -> (x+1=w245:i32)
                          n190 = local write "Seq Line Now"(w245) -> ()
                        }
                      }
                    }
                    frame "START" {
                      n191 = case shown="\"IV\"" w248 {
                        tunnel: w247 -> [w253 _]
                        tunnel: w246 -> [w249 _]
                        frame "MEASURE", Default {
                          n192 = call <vilib>:"Space Constant.vi"() -> ("String"=w254:string)
                          n193 = Match Pattern(string=w253, regular expression=w254) -> (before substring=w252:string)  [unwired: 1 in, 3 out]
                          n194 = Equal?(x=w252, y="SINGLE") -> (x = y?=w250:bool)
                          n195 = case shown="False" w250 {
                            tunnel: w249 -> [_ w270]
                            frame False {
                              n196 = flat-sequence {
                                frame #0 {
                                n197 = local write "Measure Flag"(TRUE ("Measure Flag")) -> ()
                                }
                                frame #1 {
                                n198 = local read "Measurement \nSetup"() -> (w256:u16)
                                n199 = case shown="1" w256 {
                                frame 0, Default {
                                n200 = local read "DC Pulse"() -> (w258:bool)
                                n201 = local read "6221 Address"() -> (w257:string)
                                n202 = case shown="False" w258 {
                                tunnel: w257 -> [w259 _]
                                frame False {
                                n203 = GPIB Write(0:w259, 1:"OUTPut ON" ("data")) -> ()  [unwired: 3 in, 2 out]
                                }
                                frame True {
                                }
                                }
                                }
                                frame 1 {
                                # "For AC Setup, turn on current source"
                                n204 = local read "6221 Address 2"() -> (w263:string)
                                n205 = local write "AC Flag"(TRUE ("AC Flag")) -> ()
                                n206 = GPIB Write(0:w263, 1:"SOUR:WAVE:ARM\nSOUR:WAVE:INIT" ("data")) -> ()  [unwired: 3 in, 2 out]
                                }
                                frame 2 {
                                }
                                }
                                }
                                frame #2 {
                                n207 = local read "Seq Line Now"() -> (w264:i32)
                                n208 = Wait (ms)(milliseconds to wait=u32 3000) -> ()  [unwired: 1 out]
                                n209 = Increment(x=w264) -> (x+1=w265:i32)
                                n210 = local write "Seq Line Now"(w265) -> ()
                                }
                              }
                            }
                            frame True {
                              # "SINGLE MEASUREMENTMENT USING AC SETUP"
                              n211 = local read "Serial Number"() -> (w269:i32)
                              n212 = local read "Current Filename"() -> (w273:path)
                              n213 = local read "Current StartTime"() -> (w272:timestamp)
                              n214 = local read "Current Amplitude 2"() -> (w271:string)
                              n215 = Add(x=w269, y=1) -> (x+y=w267:i32)
                              n216 = local write "Serial Number"(w267) -> ()
                              n217 = flat-sequence {
                                tunnel: w273 -> [w288]
                                tunnel: w272 -> [w287]
                                tunnel: w271 -> [w286]
                                tunnel: w270 -> [w281]
                                tunnel: w267 -> [w280]
                                frame #0 {
                                n218 = local read "SR860 Ch2 Address"() -> (w283:string)
                                n219 = local read "SR860 Ch1 Address"() -> (w285:string)
                                n220 = local read "Ch1 Enable"() -> (w284:bool)
                                n221 = local read "Ch2 Enable"() -> (w282:bool)
                                n222 = call "AC Measure Single.vi"("File Name"=w288, "Serial Number"=w280, "Start time"=w287, "PPMS Reference"=w281, "Current Amplitude"=w286, "Ch2 Enable"=w282, "SR860 Ch2 Address"=w283, "Ch1 Enable"=w284, "SR860 Ch1 Address"=w285) -> ("Datapoint Array"=w276:dbl[])  [unwired: 2 in]
                                n223 = local read "Data array"() -> (w275:dbl[][])
                                n224 = Reshape Array(w276, 1 ("dimension size"), 12 ("dimension size")) -> (w277:dbl[][])
                                n225 = Insert Into Array(array=w275, new element=w277) -> (w274:dbl[][])  [unwired: 2 in]
                                n226 = local write "Data array"(w274) -> ()
                                }
                                frame #1 {
                                n227 = local read "Seq Line Now"() -> (w290:i32)
                                n228 = Increment(x=w290) -> (x+1=w289:i32)
                                n229 = local write "Seq Line Now"(w289) -> ()
                                }
                              }
                            }
                          }
                        }
                        frame "IV" {
                          n230 = case shown="True" "IV - DC/AC" {
                            tunnel: "6221 Address - IV" -> [w335 w353]
                            tunnel: "IV Sampling" -> [w337 w349]
                            tunnel: "IV Type" -> [w336 w350]
                            tunnel: "dI or Imin" -> [w338 w348]
                            tunnel: "Imax" -> [w339 w347]
                            tunnel: "Points" -> [w340 w346]
                            tunnel: [w344 w354] -> w297
                            frame False {
                              # "AC - IV"
                              n231 = call "Measure IV AC.vi"("IV Sampling"=w337, "6221 Address"=w335, "SR860 Address"="SR860 Address - IV", "IV Type"=w336, "dI or Imin"=w338, "Imax"=w339, "Ipts"=w340, "Frequency"="Frequency - IV", "Filter BW"="Filter BW - IV", "Ch1 Harmonic"="Ch1 Harmonic - IV") -> ("Data array"=w344:dbl[][])  [unwired: 3 in, 2 out]
                            }
                            frame True {
                              # "DC - IV"
                              n232 = call "Measure IV DC.vi"("dI or Imin"=w348, "Imax"=w347, "IV Sampling"=w349, "IV Type"=w350, "6221 Address"=w353, "Ipts"=w346, "Period (s)"="DC Period (s)", "2182A Address"="2182A Address - IV", "2182A Buffer"="2182A Buffer") -> ("Data array"=w354:dbl[][])
                            }
                          }
                          "IV Data" <- w297
                          n233 = Get Date/Time In Seconds() -> (seconds since 1Jan1904=w308:timestamp)
                          n234 = Strip Path(path="IV Datafile Root") -> (stripped path=w325:path, name=w322:string)
                          n235 = Format Date/Time String(time format string (%c)="_%m%d_%H%M", seconds (now)=w308) -> (date/time string=w306:string)  [unwired: 1 in]
                          n236 = local read "Temperature setpoint"() -> (w296:dbl)
                          n237 = Number To Fractional String(number=w296, precision (6)=i16 2 ("width (-)")) -> (F-format string=w295:string)  [unwired: 2 in]
                          n238 = local read "Field Setpoint"() -> (w293:dbl)
                          n239 = local read "Theta Setpoint"() -> (w318:dbl)
                          n240 = Number To Fractional String(number=w293, precision (6)=i16 1) -> (F-format string=w292:string)  [unwired: 2 in]
                          n241 = Number To Decimal String(number=w318) -> (decimal integer string=w317:string)  [unwired: 1 in]
                          n242 = Concatenate Strings(w322, "_" ("string"), w295, "K_" ("string"), w292, "Oe_" ("string"), w317, "deg_" ("string"), w306, ".csv" ("string")) -> (w315:string)
                          n243 = Build Array("Current(A)", "Voltage(V)", "VoltageSTD(V)", "Resistance(ohm)", "ResistanceSTD(ohm)") -> (w333:string[])
                          n244 = Build Path(base path=w325, name or relative path=w315) -> (appended path=w324:path)
                          n245 = local read "Seq Line Now"() -> (w309:i32)
                          n246 = call-poly <vilib>:"Write Delimited Spreadsheet.vi"("file path (dialog if empty)"=w324, "1D data"=w333, "append to file? (new file:F)"=TRUE, "delimiter (\\t)"="," ("delimiter (\\t)")) -> ("new file path (Not A Path if cancelled)"=w311:path)  [unwired: 10 in, 1 out]
                          n247 = Increment(x=w309) -> (x+1=w310:i32)
                          n248 = call-poly <vilib>:"Write Delimited Spreadsheet.vi"("file path (dialog if empty)"=w311, "format (%.3f)"="%.5e" ("format string"), "2D data"=w297, "append to file? (new file:F)"=TRUE, "delimiter (\\t)"="," ("delimiter (\\t)")) -> ()  [unwired: 9 in, 2 out]
                          n249 = local write "Seq Line Now"(w310) -> ()
                        }
                      }
                    }
                    frame "STOP" {
                      n250 = flat-sequence {
                        frame #0 {
                          n251 = local write "Measure Flag"(FALSE ("Measure Flag")) -> ()
                        }
                        frame #1 {
                          n252 = local read "Measurement \nSetup"() -> (w356:u16)
                          n253 = case shown="1" w356 {
                            frame 0, Default {
                              n254 = local read "6221 Address"() -> (w357:string)
                              n255 = local read "DC Pulse"() -> (w358:bool)
                              n256 = case shown="False" w358 {
                                tunnel: w357 -> [w359 _]
                                frame False {
                                n257 = GPIB Write(0:w359, 1:"OUTPut OFF" ("data")) -> ()  [unwired: 3 in, 2 out]
                                }
                                frame True {
                                }
                              }
                            }
                            frame 1 {
                              # "Turn off current for AC System"
                              n258 = local read "6221 Address 2"() -> (w361:string)
                              n259 = GPIB Write(0:w361, 1:"SOUR:WAVE:ABORt" ("data")) -> ()  [unwired: 3 in, 2 out]
                            }
                            frame 2 {
                            }
                          }
                        }
                        frame #2 {
                          n260 = local read "Seq Line Now"() -> (w363:i32)
                          n261 = Wait (ms)(milliseconds to wait=u32 3000) -> ()  [unwired: 1 out]
                          n262 = Increment(x=w363) -> (x+1=w364:i32)
                          n263 = local write "Seq Line Now"(w364) -> ()
                        }
                      }
                    }
                    frame "SCAN" {
                      n264 = local read "scan_new"() -> (w371:bool)
                      n265 = case shown="False" w371 {
                        tunnel: w370 -> [_ w422]
                        tunnel: w369 -> [_ w421]
                        tunnel: w368 -> [_ w420]
                        tunnel: w367 -> [w375 _]
                        tunnel: w366 -> [w372 _]
                        frame False {
                          # "Not a new SCAN. Just go through the existing scan by setting the appropriate ENV"
                          n266 = local read "scan_points"() -> (w378:dbl[])
                          n267 = local read "scan_counter"() -> (w377:i16)
                          n268 = local read "scan_RATE"() -> (w374:dbl)
                          n269 = local read "scan_env"() -> (w373:string)
                          n270 = Index Array(array=w378, index=w377) -> (element=w376:dbl)
                          n271 = flat-sequence {
                            tunnel: w373 -> [w383]
                            tunnel: w372 -> [w382]
                            tunnel: w375 -> [w381]
                            tunnel: w376 -> [w380]
                            tunnel: w374 -> [w379]
                            frame #0 {
                              n272 = case shown="\"CURRENT\"" w383 {
                                tunnel: w382 -> [w384 _ _ _ _]
                                tunnel: w381 -> [_ w391 w394 w397 _]
                                tunnel: w380 -> [_ w389 w393 w396 w401]
                                tunnel: w379 -> [_ w390 w395 w398 _]
                                frame "INVALID", Default {
                                n273 = Number To Decimal String(number=w384) -> (decimal integer string=w386:string)  [unwired: 1 in]
                                n274 = Concatenate Strings("Invalid Environment Variable encountered on line " ("string"), w386) -> (w385:string)
                                n275 = call "Display Message to User3"("Enable"=TRUE, "Message"=w385) -> ()  [unwired: 8 in, 2 out]
                                }
                                frame "TEMP" {
                                w392 = 0 items=["FastSettle", "NoOvershoot"] ("Approach")
                                n276 = call "SetTemperature.vi"("Approach"=w392, "Rate"=w390, "Temperature"=w389, "Instrument Ref In"=w391) -> ()  [unwired: 3 in, 3 out]
                                n277 = local write "Temperature setpoint"(w389) -> ()
                                }
                                frame "FIELD" {
                                n278 = call "SetField.vi"("Rate"=w395, "Field"=w393, "Instrument Ref In"=w394) -> ()  [unwired: 4 in, 3 out]
                                n279 = local write "Field Setpoint"(w393) -> ()
                                }
                                frame "THETA" {
                                n280 = local write "Theta Setpoint"(w396) -> ()
                                n281 = call "SetPosition.vi"("Speed"=w398, "Position"=w396, "Instrument Ref In"=w397) -> ()  [unwired: 4 in, 3 out]
                                }
                                frame "CURRENT" {
                                n282 = local read "Measurement \nSetup"() -> (w399:u16)
                                n283 = Number To Exponential String(number=w401) -> (E-format string=w400:string)  [unwired: 3 in]
                                n284 = case shown="0, Default" w399 {
                                tunnel: w400 -> [w402 w413]
                                frame 0, Default {
                                n285 = local read "6221 Address"() -> (w404:string)
                                n286 = local write "Current Amplitude"(w402) -> ()
                                n287 = local read "DC Pulse"() -> (w403:bool)
                                n288 = case shown="True" w403 {
                                tunnel: w404 -> [w407 w410]
                                tunnel: w402 -> [w405 w411]
                                frame False {
                                n289 = Concatenate Strings("CURRent ", w405) -> (w406:string)
                                n290 = GPIB Write(0:w407, 1:w406) -> ()  [unwired: 3 in, 2 out]
                                }
                                frame True {
                                n291 = Concatenate Strings("SOUR:WAVE:AMPL " ("string"), w411) -> (w412:string)
                                n292 = GPIB Write(0:w410, 1:w412) -> ()  [unwired: 3 in, 2 out]
                                }
                                }
                                }
                                frame 1 {
                                n293 = local read "6221 Address 2"() -> (w414:string)
                                n294 = local write "Current Amplitude 2"(w413) -> ()
                                n295 = Concatenate Strings("SOUR:WAVE:AMPL " ("string"), w413) -> (w416:string)
                                n296 = GPIB Write(0:w414, 1:w416) -> ()  [unwired: 3 in, 2 out]
                                }
                                }
                                }
                              }
                            }
                            frame #1 {
                              n297 = local read "Seq Line Now"() -> (w417:i32)
                              n298 = Increment(x=w417) -> (x+1=w418:i32)
                              n299 = local write "Seq Line Now"(w418) -> ()
                              n300 = Wait (ms)(milliseconds to wait=u32 3000) -> ()  [unwired: 1 out]
                            }
                          }
                        }
                        frame True {
                          # "New SCAN just started"
                          n301 = flat-sequence {
                            tunnel: w422 -> [w424]
                            tunnel: w421 -> [w437]
                            tunnel: w420 -> [w426]
                            frame #0 {
                              n302 = local write "scan_head"(w424) -> ()
                              n303 = local write "scan_new"(FALSE ("scan_new")) -> ()
                            }
                            frame #1 {
                              w436 = 0 ("index (row)")
                              n304 = Index Array(array=w437, index (row)=w436) -> (element=w432:dbl[])  [unwired: 1 in]
                              n305 = Index Array(array=w437, index (row)=w436) -> (element=w433:dbl[])  [unwired: 1 in]
                              n306 = Index Array(array=w437, index (row)=w436) -> (element=w434:dbl[])  [unwired: 1 in]
                              n307 = Index Array(array=w437, index (row)=w436) -> (element=w435:dbl[])  [unwired: 1 in]
                              n308 = Index Array(array=w432, index=4) -> (element=w431:dbl)
                              n309 = Index Array(array=w433, index=2) -> (element=w425:dbl)
                              n310 = Index Array(array=w434, index=1) -> (element=w428:dbl)
                              n311 = Index Array(array=w435, index=0) -> (element=w429:dbl)
                              n312 = local write "scan_RATE"(w431) -> ()
                              n313 = local write "scan_npts"(w425) -> ()
                              n314 = call-poly <vilib>:"Ramp Pattern.vi"("exclude end?"=FALSE, "start"=w429, "end"=w428, "samples"=w425) -> ("Ramp Pattern"=w427:dbl[])  [unwired: 6 in, 1 out]
                              n315 = local write "scan_env"(w426) -> ()
                              n316 = local write "scan_points"(w427) -> ()
                            }
                            frame #2 {
                              n317 = local read "scan_head"() -> (w442:i32)
                              n318 = local write "Seq Line Now"(w442) -> ()
                              n319 = local write "scan_counter"(i16 0 ("scan_counter")) -> ()
                            }
                          }
                        }
                      }
                    }
                    frame "END" {
                      # "Check if SCAN endpoint reached"
                      n320 = Index Array(array=w448, index (row)=0) -> (element=w449:dbl[])  [unwired: 1 in]
                      n321 = local read "scan_counter"() -> (w447:i16)
                      n322 = Index Array(array=w449, index=2) -> ()  [unwired: 1 out]
                      n323 = Decrement(x="scan_npts") -> (x-1=w444:i16)
                      n324 = Less?(x=w447, y=w444) -> (x < y?=w445:bool)
                      n325 = case shown="False" w445 {
                        frame False {
                          # "SCAN endpoint reached.\nJust move SET the scan_new flag and move on to the next line"
                          n326 = local write "scan_new"(TRUE ("scan_new")) -> ()
                          n327 = local read "Seq Line Now"() -> (w453:i32)
                          n328 = Increment(x=w453) -> (x+1=w452:i32)
                          n329 = local write "Seq Line Now"(w452) -> ()
                        }
                        frame True {
                          # "Increment scan_counter\nChange SeqLineNow to scan_head"
                          # "SCAN endpoint not reached yet"
                          n330 = local read "scan_counter"() -> (w456:i16)
                          n331 = Increment(x=w456) -> (x+1=w457:i16)
                          n332 = local write "scan_counter"(w457) -> ()
                          n333 = local read "scan_head"() -> (w455:i32)
                          n334 = local write "Seq Line Now"(w455) -> ()
                        }
                      }
                    }
                    frame "NEWFILE" {
                      n335 = local read "Datafile Path"() -> (w470:path)
                      n336 = Strip Path(path=w470) -> (stripped path=w469:path)  [unwired: 1 out]
                      n337 = Build Path(base path=w469, name or relative path=w468) -> (appended path=w467:path)
                      n338 = local write "Datafile Path"(w467) -> ()
                      n339 = call "Create New Datafile.vi"("Metadata"="Metadata", "Filetype"="Filetype", "File Base"=w467) -> ("Start time"=w464:timestamp, "File name"=w465:path)
                      n340 = local write "Current Filename"(w465) -> ()
                      n341 = local write "Current StartTime"(w464) -> ()
                      n342 = local write "Time Elasped"(0.0 ("Time Elasped")) -> ()
                      n343 = local write "Serial Number"(0) -> ()
                      n344 = local write "Data array"(dbl[][] [] ("Data array")) -> ()
                      n345 = local read "Seq Line Now"() -> (w458:i32)
                      n346 = Increment(x=w458) -> (x+1=w459:i32)
                      n347 = local write "Seq Line Now"(w459) -> ()
                    }
                    frame "#", Default {
                      # "Let go. This is considered a comment"
                      n348 = local read "Seq Line Now"() -> (w471:i32)
                      n349 = Increment(x=w471) -> (x+1=w472:i32)
                      n350 = local write "Seq Line Now"(w472) -> ()
                    }
                    frame "" {
                      # "Blank line disregarded as a comment"
                      n351 = local read "Seq Line Now"() -> (w473:i32)
                      n352 = Increment(x=w473) -> (x+1=w474:i32)
                      n353 = local write "Seq Line Now"(w474) -> ()
                    }
                    frame "SET" {
                      n354 = Index Array(array=w483, index (row)=0) -> (element=w482:dbl[])  [unwired: 1 in]
                      n355 = Index Array(array=w483, index (row)=0) -> (element=w481:dbl[])  [unwired: 1 in]
                      n356 = Index Array(array=w482, index=0) -> (element=w477:dbl)
                      n357 = Index Array(array=w481, index=2) -> (element=w476:dbl)
                      n358 = local write "SET Rate"(w476) -> ()
                      n359 = local write "SET Setpoint"(w477) -> ()
                      n360 = flat-sequence {
                        tunnel: w480 -> [w491]
                        tunnel: w479 -> [w490]
                        tunnel: w478 -> [w489]
                        tunnel: w477 -> [w488]
                        tunnel: w476 -> [w487]
                        frame #0 {
                          n361 = case shown="\"THETA\"" w491 {
                            tunnel: w490 -> [w492 _ _ _ _ _]
                            tunnel: w489 -> [_ w499 w502 w505 _ _]
                            tunnel: w488 -> [_ w497 w501 w504 w509 _]
                            tunnel: w487 -> [_ w498 w503 w506 _ _]
                            frame "INVALID", Default {
                              n362 = Number To Decimal String(number=w492) -> (decimal integer string=w494:string)  [unwired: 1 in]
                              n363 = Concatenate Strings("Invalid Environment Variable encountered on line " ("string"), w494) -> (w493:string)
                              n364 = call "Display Message to User"("Enable"=TRUE, "Message"=w493) -> ()  [unwired: 8 in, 2 out]
                            }
                            frame "TEMP" {
                              w500 = 0 items=["FastSettle", "NoOvershoot"] ("Approach")
                              n365 = call "SetTemperature.vi"("Approach"=w500, "Rate"=w498, "Temperature"=w497, "Instrument Ref In"=w499) -> ()  [unwired: 3 in, 3 out]
                              n366 = local write "Temperature setpoint"(w497) -> ()
                            }
                            frame "FIELD" {
                              n367 = call "SetField.vi"("Rate"=w503, "Field"=w501, "Instrument Ref In"=w502) -> ()  [unwired: 4 in, 3 out]
                              n368 = local write "Field Setpoint"(w501) -> ()
                            }
                            frame "THETA" {
                              n369 = local write "Theta Setpoint"(w504) -> ()
                              n370 = call "SetPosition.vi"("Speed"=w506, "Position"=w504, "Instrument Ref In"=w505) -> ()  [unwired: 4 in, 3 out]
                            }
                            frame "CURRENT" {
                              n371 = local read "Measurement \nSetup"() -> (w507:u16)
                              n372 = Number To Exponential String(number=w509) -> (E-format string=w508:string)  [unwired: 3 in]
                              n373 = case shown="1" w507 {
                                tunnel: w508 -> [w510 w521]
                                frame 0, Default {
                                n374 = local read "6221 Address"() -> (w512:string)
                                n375 = local write "Current Amplitude"(w510) -> ()
                                n376 = local read "DC Pulse"() -> (w511:bool)
                                n377 = case shown="True" w511 {
                                tunnel: w512 -> [w515 w518]
                                tunnel: w510 -> [w513 w519]
                                frame False {
                                n378 = Concatenate Strings("CURRent ", w513) -> (w514:string)
                                n379 = GPIB Write(0:w515, 1:w514) -> ()  [unwired: 3 in, 2 out]
                                }
                                frame True {
                                n380 = Concatenate Strings("SOUR:WAVE:AMPL " ("string"), w519) -> (w520:string)
                                n381 = GPIB Write(0:w518, 1:w520) -> ()  [unwired: 3 in, 2 out]
                                }
                                }
                                }
                                frame 1 {
                                n382 = local read "6221 Address 2"() -> (w522:string)
                                n383 = local write "Current Amplitude 2"(w521) -> ()
                                n384 = Concatenate Strings("SOUR:WAVE:AMPL " ("string"), w521) -> (w524:string)
                                n385 = GPIB Write(0:w522, 1:w524) -> ()  [unwired: 3 in, 2 out]
                                }
                              }
                            }
                            frame "AC-SINGLE" {
                              n386 = flat-sequence {
                                tunnel: [w531] -> w526
                                tunnel: [w530] -> w525
                                tunnel: w526 -> [w536]
                                tunnel: w525 -> [w535]
                                frame #0 {
                                n387 = local read "6221 Address 2"() -> (w528:string)
                                n388 = Wait (ms)(milliseconds to wait=u32 1000) -> ()  [unwired: 1 out]
                                n389 = GPIB Write(0:w528, 1:"SOUR:WAVE:ARM\nSOUR:WAVE:INIT" ("data")) -> ()  [unwired: 3 in, 2 out]
                                }
                                frame #1 {
                                w532 = "CAPTURELEN 8;\nARNG;\nASCL;" ("data")
                                n390 = local read "SR860 Ch1 Address"() -> (w531:string)
                                n391 = local read "SR860 Ch2 Address"() -> (w530:string)
                                n392 = GPIB Write(0:w530, 1:w532) -> ()  [unwired: 3 in, 2 out]
                                n393 = GPIB Write(0:w531, 1:w532) -> ()  [unwired: 3 in, 2 out]
                                n394 = Wait (ms)(milliseconds to wait=u32 1500) -> ()  [unwired: 1 out]
                                }
                                frame #2 {
                                w537 = "APHS;" ("data")
                                n395 = GPIB Write(0:w535, 1:w537) -> ()  [unwired: 3 in, 2 out]
                                n396 = GPIB Write(0:w536, 1:w537) -> ()  [unwired: 3 in, 2 out]
                                n397 = Wait (ms)(milliseconds to wait=u32 3500) -> ()  [unwired: 1 out]
                                }
                              }
                            }
                          }
                        }
                        frame #1 {
                          n398 = local read "Seq Line Now"() -> (w538:i32)
                          n399 = Increment(x=w538) -> (x+1=w539:i32)
                          n400 = local write "Seq Line Now"(w539) -> ()
                          n401 = Wait (ms)(milliseconds to wait=u32 3000) -> ()  [unwired: 1 out]
                        }
                      }
                    }
                  }
                  "Command" <- w183
                  "Current Line" <- w184
                  "ENV VAR" <- w181
                  "Parameters" <- w182
                  "Current Line Number" <- w179
                }
              }
              n402 = And(x=w157, y=w156) -> (x .and. y?=w158:bool)
              n403 = Not(x=w158) -> (.not. x?=w162:bool)
            }
          }
          frame #2 {
            n404 = local write "ExecSeq"(FALSE ("ExecSeq")) -> ()
          }
        }
      }
    }
    n405 = local read "STOP Flag"() -> (w140:bool)
  }
  n406 = while {
    tunnel: w4 -> [w542]
    stop <- w543 stop-if-true
    n407 = local read "Measure Flag"() -> (w544:bool)
    n408 = case shown="True" w544 {
      tunnel: w542 -> [_ w547]
      frame False {
        n409 = Wait (ms)(milliseconds to wait=u32 100) -> ()  [unwired: 1 out]
      }
      frame True {
        n410 = stacked-sequence {
          frame #0 {
            n411 = Wait (ms)(milliseconds to wait=u32 500) -> ()  [unwired: 1 out]
            "Measure Blink" <- TRUE ("Initialised")
          }
          frame #1 {
            n412 = local write "Measure Blink"(FALSE ("Measure Blink")) -> ()
            n413 = Wait (ms)(milliseconds to wait=u32 500) -> ()  [unwired: 1 out]
          }
        }
        n414 = local read "Measurement \nSetup"() -> (w546:u16)
        n415 = stacked-sequence {
          seq-local: [w557 _] -> [_ w664]
          seq-local: [w554 _] -> [_ w661]
          seq-local: [w553 _] -> [_ w662]
          seq-local: [w558 _] -> [_ w665]
          seq-local: [w559 _] -> [_ w666]
          seq-local: [w552 _] -> [_ w663]
          seq-local: [w556 _] -> [_ w659]
          seq-local: [w555 _] -> [_ w660]
          seq-local: [w549 _] -> [_ w657]
          seq-local: [w548 _] -> [_ w656]
          tunnel: w547 -> [w551 _]
          tunnel: w546 -> [w550 _]
          frame #0 {
            n416 = stacked-sequence {
              tunnel: w550 -> [_ w590]
              tunnel: [_ w595] -> w556
              tunnel: [_ w594] -> w555
              tunnel: [_ w593] -> w554
              tunnel: [_ w592] -> w553
              tunnel: [_ w591] -> w552
              tunnel: [_ w589] -> w549
              tunnel: [_ w588] -> w548
              frame #0 {
                # "If the flag is ON,\nwe wait for 5s to allow\nthe lock-in and current \nsource to settle.\nThen we turn off the flag\nto not do this again.\nThen we proceed to \nmeasurements."
                # "AC Flag is turned ON if\n- AC Current source of turned ON - inside sequence or with \"Measure Device\" button"
                n417 = local read "AC Flag"() -> (w560:bool)
                n418 = case shown="True" w560 {
                  frame False {
                  }
                  frame True {
                    n419 = stacked-sequence {
                      seq-local: [_ w566 _ _] -> [_ _ w581 _]
                      seq-local: [_ w564 _ _] -> [_ _ w580 _]
                      seq-local: [_ w563 _ _] -> [_ _ w579 _]
                      seq-local: [_ w562 _ _] -> [_ _ w578 _]
                      frame #0 {
                        n420 = Wait (ms)(milliseconds to wait=u32 1000) -> ()  [unwired: 1 out]
                      }
                      frame #1 {
                        w565 = "ARNG;\nASCL;" ("data")
                        n421 = local read "SR860 Ch2 Address"() -> (w562:string)
                        n422 = local read "Ch2 Enable"() -> (w563:bool)
                        n423 = local read "Ch1 Enable"() -> (w564:bool)
                        n424 = local read "SR860 Ch1 Address"() -> (w566:string)
                        n425 = case shown="True" w563 {
                          tunnel: w565 -> [_ w569]
                          tunnel: w562 -> [_ w568]
                          frame False {
                          }
                          frame True {
                            n426 = GPIB Write(0:w568, 1:w569) -> ()  [unwired: 3 in, 2 out]
                          }
                        }
                        n427 = case shown="True" w564 {
                          tunnel: w565 -> [_ w571]
                          tunnel: w566 -> [_ w570]
                          frame False {
                          }
                          frame True {
                            n428 = GPIB Write(0:w570, 1:w571) -> ()  [unwired: 3 in, 2 out]
                          }
                        }
                        n429 = Wait (ms)(milliseconds to wait=u32 1500) -> ()  [unwired: 1 out]
                      }
                      frame #2 {
                        n430 = local read "Buffer Size (kB)"() -> (w577:i32)
                        n431 = Number To Decimal String(number=w577) -> (decimal integer string=w574:string)  [unwired: 1 in]
                        n432 = Concatenate Strings("CAPTURELEN " ("data"), w574, ";" ("string"), "APHS;" ("data")) -> (w572:string)
                        n433 = case shown="True" w579 {
                          tunnel: w572 -> [_ w584]
                          tunnel: w578 -> [_ w583]
                          frame False {
                          }
                          frame True {
                            n434 = GPIB Write(0:w583, 1:w584) -> ()  [unwired: 3 in, 2 out]
                          }
                        }
                        n435 = case shown="True" w580 {
                          tunnel: w581 -> [_ w586]
                          tunnel: w572 -> [_ w585]
                          frame False {
                          }
                          frame True {
                            n436 = GPIB Write(0:w586, 1:w585) -> ()  [unwired: 3 in, 2 out]
                          }
                        }
                        n437 = Wait (ms)(milliseconds to wait=u32 3500) -> ()  [unwired: 1 out]
                      }
                      frame #3 {
                        n438 = local write "AC Flag"(FALSE ("AC Flag")) -> ()
                      }
                    }
                  }
                }
              }
              frame #1 {
                n439 = case shown="0, Default" w590 {
                  tunnel: [w610 w635] -> w595
                  tunnel: [w609 w636] -> w594
                  tunnel: [w608 w637] -> w593
                  tunnel: [w607 w638] -> w592
                  tunnel: [w598 w643] -> w591
                  tunnel: [w596 w634] -> w589
                  tunnel: [w596 w633] -> w588
                  frame 0, Default {
                    w596 = nan
                    # "DC System"
                    n440 = local read "Voltmeter 2 Address"() -> (w600:string)
                    n441 = local read "Voltmeter 1 Address"() -> (w601:string)
                    n442 = local read "Current Amplitude"() -> (w599:string)
                    n443 = local read "Time Period (s)"() -> (w603:string)
                    n444 = local read "6221 Address"() -> (w602:string)
                    n445 = local read "Channel 1"() -> (w605:bool)
                    n446 = local read "Channel 2"() -> (w606:bool)
                    n447 = local read "Tpad(ms)"() -> (w604:i32)
                    n448 = local read "DC Pulse"() -> (w597:bool)
                    n449 = case shown="True" w597 {
                      tunnel: [w620 w632] -> w610
                      tunnel: [w619 w631] -> w609
                      tunnel: [w618 w630] -> w608
                      tunnel: [w617 w629] -> w607
                      tunnel: w606 -> [w611 w628]
                      tunnel: w605 -> [w612 w627]
                      tunnel: w604 -> [_ w626]
                      tunnel: w603 -> [w613 w625]
                      tunnel: w602 -> [_ w624]
                      tunnel: w601 -> [w615 w623]
                      tunnel: w600 -> [w616 w622]
                      tunnel: w599 -> [w614 w621]
                      frame False {
                        n450 = call "DC Basic Measure.vi"("Channel 2"=w611, "Voltmeter 2 Address"=w616, "Channel 1"=w612, "Voltmeter 1 Address"=w615, "Period (s)"=w613, "Amplitude (A)"=w614) -> ("STD 2"=w617:dbl, "Resistance 2"=w618:dbl, "STD 1"=w619:dbl, "Resistance 1"=w620:dbl)  [unwired: 2 in]
                      }
                      frame True {
                        n451 = call "DC Transport Measure.vi"("Channel 2"=w628, "Voltmeter 2 Address"=w622, "Channel 1"=w627, "Voltmeter 1 Address"=w623, "tpad"=w626, "Period (s)"=w625, "Amplitude (A)"=w621, "6221 Address"=w624) -> ("STD 2"=w629:dbl, "Resistance 2"=w630:dbl, "STD 1"=w631:dbl, "Resistance 1"=w632:dbl)
                      }
                    }
                    n452 = Fract/Exp String To Number(string=w599) -> (number=w598:dbl)  [unwired: 3 in, 1 out]
                  }
                  frame 1 {
                    # "AC System"
                    n453 = local read "Buffer Offset (kb)"() -> (w647:string)
                    n454 = local read "Buffer Size (kB)"() -> (w646:i32)
                    n455 = local read "Ch1 Enable"() -> (w648:bool)
                    n456 = local read "Ch2 Enable"() -> (w645:bool)
                    n457 = local read "SR860 Ch1 Address"() -> (w649:string)
                    n458 = local read "SR860 Ch2 Address"() -> (w644:string)
                    n459 = local read "Current Amplitude 2"() -> (w650:string)
                    n460 = Fract/Exp String To Number(string=w650) -> (number=w643:dbl)  [unwired: 3 in, 1 out]
                    n461 = call "AC Transport Measure.vi"("SR860 Ch1 Address"=w649, "Ch1 Enable"=w648, "Buffer Offset (kb)"=w647, "Buffer Size (kb)"=w646, "Ch2 Enable"=w645, "SR860 Ch2 Address"=w644) -> ("R1 Mean"=w642:dbl, "R2 Mean"=w640:dbl, "R1 STD"=w641:dbl, "T1 Mean"=w634:dbl, "T2 Mean"=w633:dbl, "R2 STD"=w639:dbl)  [unwired: 6 in, 2 out]
                    n462 = Divide(x=w642, y=w643) -> (x/y=w635:dbl)
                    n463 = Divide(x=w641, y=w643) -> (x/y=w636:dbl)
                    n464 = Divide(x=w640, y=w643) -> (x/y=w637:dbl)
                    n465 = Divide(x=w639, y=w643) -> (x/y=w638:dbl)
                  }
                }
              }
            }
            n466 = stacked-sequence {
              tunnel: [_ w655] -> w559
              tunnel: [_ w654] -> w558
              tunnel: [_ w653] -> w557
              tunnel: w551 -> [_ w652]
              frame #0 {
                n467 = Wait (ms)(milliseconds to wait=u32 500) -> ()  [unwired: 1 out]
              }
              frame #1 {
                # "Get PPMS Status\nin the middle of the \ntransport measurement"
                n468 = call "Get All Status.vi"("Instrument Ref In"=w652) -> ("Field"=w654:dbl, "Temperature"=w655:dbl, "Position"=w653:dbl)  [unwired: 3 in, 5 out]
              }
            }
          }
          frame #1 {
            # "Check measure flag before accumulating data as measure flag might've been turned off during the measurement period\nSuch a measurement is often garbage"
            n469 = local read "Serial Number"() -> (w671:i32)
            n470 = local read "Current StartTime"() -> (w667:timestamp)
            n471 = local read "Current Filename"() -> (w669:path)
            n472 = local read "Measure Flag"() -> (w658:bool)
            n473 = Add(x=w671, y=1) -> (x+y=w668:i32)
            n474 = local write "Serial Number"(w668) -> ()
            n475 = case shown="True" w658 {
              tunnel: w669 -> [_ w687]
              tunnel: w668 -> [_ w686]
              tunnel: w667 -> [_ w685]
              tunnel: w666 -> [_ w684]
              tunnel: w665 -> [_ w683]
              tunnel: w664 -> [_ w682]
              tunnel: w663 -> [_ w679]
              tunnel: w662 -> [_ w678]
              tunnel: w661 -> [_ w677]
              tunnel: w660 -> [_ w676]
              tunnel: w659 -> [_ w675]
              tunnel: w657 -> [_ w673]
              tunnel: w656 -> [_ w672]
              frame False {
              }
              frame True {
                n476 = local read "ExecSeq"() -> (w674:bool)
                n477 = case shown="True" w674 {
                  tunnel: w687 -> [_ w720]
                  tunnel: w686 -> [w706 w719]
                  tunnel: w685 -> [w705 w718]
                  tunnel: w684 -> [w703 w717]
                  tunnel: w683 -> [w702 w716]
                  tunnel: w682 -> [w701 w715]
                  tunnel: [w700 w714] -> w681
                  tunnel: w679 -> [w699 w713]
                  tunnel: w678 -> [w695 w712]
                  tunnel: w677 -> [w696 w711]
                  tunnel: w676 -> [w697 w710]
                  tunnel: w675 -> [w698 w709]
                  tunnel: w673 -> [w693 w708]
                  tunnel: w672 -> [w692 w707]
                  frame False {
                    n478 = Get Date/Time In Seconds() -> (seconds since 1Jan1904=w694:timestamp)
                    n479 = Subtract(x=w694, y=w705) -> (x-y=w704:dbl)
                    n480 = Build Array(w706, w704, w703, w702, w701, w699, w698, w697, w696, w695, w693, w692) -> (w700:dbl[])
                  }
                  frame True {
                    n481 = call "Create Datafile Entry.vi"("Serial Number"=w719, "Resistance 1"=w709, "STD 1"=w710, "File Name"=w720, "Phase 1"=w708, "Start time"=w718, "Phase 2"=w707, "Temperature"=w717, "Field"=w716, "Theta"=w715, "Resistance 2"=w711, "STD 2"=w712, "Current Level"=w713) -> ("Datapoint Array"=w714:dbl[])  [unwired: 2 in]
                  }
                }
                n482 = Reshape Array(w681, 1 ("dimension size"), 12 ("dimension size")) -> (w680:dbl[][])
                n483 = local read "Data array"() -> (w689:dbl[][])
                n484 = Insert Into Array(array=w689, new element=w680) -> (w688:dbl[][])  [unwired: 2 in]
                n485 = local write "Data array"(w688) -> ()
              }
            }
          }
        }
      }
    }
    n486 = local read "STOP Flag"() -> (w543:bool)
  }
  "Initialised" <- FALSE ("Initialised")
  "Measure Flag" <- FALSE ("Measure Flag")
  "ExecSeq" <- FALSE ("Initialised")
  "STOP Flag" <- FALSE ("Initialised")
  "AC Flag" <- FALSE ("AC Current Flag")
  "scan_new" <- TRUE ("scan_new")
